vi "Striptest.vi"(1 "Simulation?":bool) -> ()   [LabVIEW 2018]
uses:
  general_VIs/globals/QC_RunInformation.vi
  striptest/ProbePlan/ProbePlanParams.vi
  InstrControl/SupplyControl/SupplyControl.lvclass
  <vilib>/regexp/Match Regular Expression.xnode
  InstrControl/InstrumentSetup.vi
  InstrControl/InstrControl.lvclass
  InstrControl/ArduinoControl/ArduinoControl.lvclass
  general_VIs/globals/QC_MeasurementSetup.vi
  InstrControl/Switching/Switching.lvclass
  InstrControl/ProbeStationControl/ProbeStationControl.lvclass
  <vilib>/Analysis/NI_AALBase.lvlib
  InstrControl/LCRControl/LCRControl.lvclass
panel:
  out "Resistance [MW]":cluster{u32, i32, "Array OUT":dbl[]}(graph)
  out "Tab Control":enum32{"Striptest Setup", "Striptest"}(tab)
  in  "Length1":dbl=2.386 caption="Length [cm]"
  in  "Length2":dbl=2.386
  in  "Length3":dbl=2.386
  in  "Length4":dbl=2.386
  in  "Bias Voltage [V]":dbl=-150.0 format="%.1f"
  in  "Frequency [Hz] Setup":i32=1000 caption="Frequency [Hz]" format="%#.3p"
  in  "Minimum fraction\nof good strips":dbl=98.0 format="%.1g"
  in  "Quit":bool
  in  "Continue":bool
  in  "Measurement Configurations":bool
  in  "Pinholes Y/N":bool=TRUE
  in  "Capacitance Y/N":bool=TRUE
  in  "Resistance Y/N":bool=TRUE
  in  "Striptest SMU":string(combo)="Keithley 2410"
  in  "LCR Meter":string(combo)="WayneKerr 6440B"
  in  "Temperature":enum16{"Read Arduino", "Enter manually"}(ring)
  in  "Bias Supply":string(combo)="Keithley 2410"
  in  "Hardware Configurations":bool
  in  "DB Serial No. IN:":string caption="DB Serial No.:"
  in  "User:":string(combo)="Christoph"
  in  "Batch No. IN:":string caption="Batch No.:"
  in  "Device Category IN:":string(combo)="Short Strip" caption="Device Category:"
  in  "Wafer No. IN:":string caption="Wafer No.:"
  in  "From4":u16(ring)
  in  "From3":u16(ring)
  in  "From2":u16(ring)
  in  "From 1":u16(ring) caption="From"
  in  "To4":u16(ring)
  in  "To3":u16(ring)
  in  "To2":u16(ring)
  in  "To 1":u16(ring) caption="To"
  out "Region 1":string caption="Region"
  out "Region2":string
  out "Region3":string
  out "Region4":string
  in  "Enable1":bool
  in  "Enable4":bool
  in  "Enable2":bool
  in  "Enable3":bool
  in  "Pinhole Parameters IN":T1={"Base Voltage"=10.0, "Base Ramp [V/step]"=10.0, "Base Step [ms]"=1000, "High Voltage"=100.0, "High Ramp [V/step]"=100.0, "High Step [ms]"=1000} caption="Pinhole Measurement Parameters"
  in  "Manufacturer:":string(combo)="Hamamatsu"
  in  "Auto ReCheck":bool
  in  "Thresholds:":T2={"Current [nA]"=200.0, "Ccoupl Lo [pF/cm]"=20.0, "Ccoupl Hi [pF/cm]"=33.0, "Rbias Lo [MW]"=1.0, "Rbias Hi [MW]"=2.0}
  in  "Rolling\nCurrent Readout":bool=TRUE
  in  "settling\ndelay [ms]":i32=50
  in  "Pinhole Parameters":T1={"Base Voltage"=10.0, "Base Ramp [V/step]"=10.0, "Base Step [ms]"=1000, "High Voltage"=100.0, "High Ramp [V/step]"=100.0, "High Step [ms]"=1000}
  out "Bias On/Off:":bool
  in  "Auto quit &\nswitch off bias":bool
  out "Sensor No.:":string
  out "Device Category:":string
  out "DB Serial No.:":string
  out "Initiated:":string
  in  "ReCheck":bool
  in  "Save Data":bool
  in  "Abort":bool
  in  "Quit w/o saving":bool
  out "Probing Region:":string
  out "Probe Point:":string
  out "Current [nA]:":dbl format="%#.2g"
  out "Capacitance [pF]:":dbl format="%#.2g"
  out "Reistance [MW]:":dbl format="%#.3g"
  out "Last Probe at:":string
  out "Run Duration:":string
  out "Estimated Completion:":string
  out "Status:":string
  out "Probe Card Channels":i32=32
  in  "Show:":u16(ring) items=["Segment4"]
  out "Defects":i32[][](graph)
  out "% OK:":dbl
  out "# total defects:":i32
  out "# probed":i32
  out "Bad Strip List":i32[](array[numeric])
  out "defect type array":i32[](array[numeric])
  out "Capacitance [pF]":cluster{u32, i32, "Array OUT":dbl[]}(graph)
  out "Current [nA]":cluster{u32, i32, "Array OUT":dbl[]}(graph)
  out "Current Reference 100V":dbl[](array[numeric])
  out "Current Reference 10V":dbl[](array[numeric])
  out "Single Needle":bool
  out "Z profile":i32[][](array[numeric])
  out "Start Temperature [°C]":dbl
  out "Last Temperature [°C]":dbl
  out "disabled channels":i32[](array[numeric])
  out "Module failed/passed":bool
  out "min scale array":i32[](array[numeric])
  out "max scale array":i32[](array[numeric])
  out "total strip number":u32
  out "Region Indices":i32[](array[numeric])
  out "Current Bias Voltage [V]":dbl
  out "Temperature Progression":T3
  out "probe points per region":i32[](array[numeric])
  # "Sensor QC: Striptest"
  # "University of \nCambridge"
  # "Current [nA]"
  # "Statistical information:"
  # "Pinholes:"
  # "Capacitance [pF]"
  # "Punchthroughs:"
  # "Shorts:"
  # "Opens:"
  # "Rpoly:"
  # "Resistance [MW]"
  # "Implant:"
  # "Current segment:"
  # "Ok  Pinhole at base  Pinhole after ramp  Short  Open  Rbias"
  # "Probe Range"
  # "Measurement Configuration"
  # "Hardware"
  # "DUT Description"
  # "Tests Included"
  # "Current status:"
  # "Measurement parameters:"
  # "DUT & Test Description:"
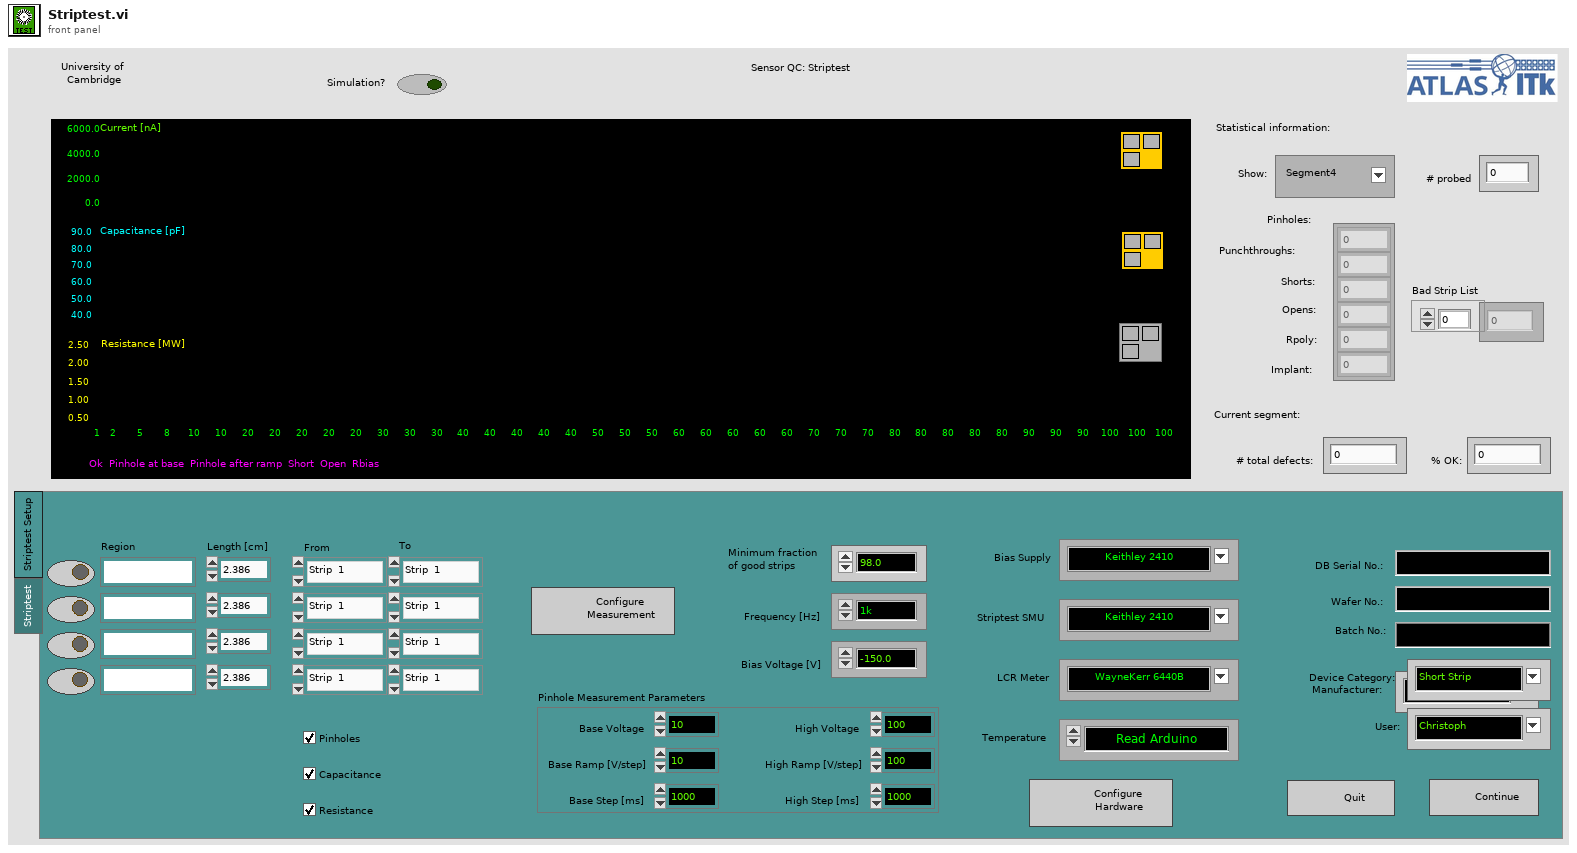
[diagram p1: front panel]
types:
  T1 = cluster{"Base Voltage":dbl, "Base Ramp [V/step]":dbl, "Base Step [ms]":i32, "High Voltage":dbl, "High Ramp [V/step]":dbl, "High Step [ms]":i32}
  T2 = cluster{"Current [nA]":dbl, "Ccoupl Lo [pF/cm]":dbl, "Ccoupl Hi [pF/cm]":dbl, "Rbias Lo [MW]":dbl, "Rbias Hi [MW]":dbl}
  T3 = cluster{"Time Array":string[], "Temperature Array [°C]":dbl[], "Humidity Array [RH %]":dbl[]}
  T4 = enum16{"Supply", "LCR", "Multimeter", "Switching"}
  T5 = enum16{"Reset", "Read Array", "Read Element", "Write Element", "Write Array", "Add Element", "Add Array"}
  T6 = enum16{"Reset", "Ground", "Striptest SMU", "Striptest LCR", "IV", "CV", "Interstrip Cap", "Interstrip Res"}
  T7 = enum16{"Reference measurement", "Baseline correcetion 10V", "Baseline correcetion 100V", "Nothing"}
  T8 = cluster{"Bias Supply":refnum<class "SupplyControl.lvclass">, "SMU":refnum<class "SupplyControl.lvclass">, "LCR":refnum<class "LCRControl.lvclass">, "ProbeStation":refnum<class "ProbeStationControl.lvclass">, "Arduino":refnum<class "ArduinoControl.lvclass">, "Measurement switch":refnum<class "Switching.lvclass">, "Probe Card Channels":i32, "Bias Voltage [V]":dbl, "First strip":i32, "Last strip":i32, "Base Voltage [V]":dbl, "Base Ramp Step [V]":dbl, "Base Ramp Interval [ms]":u32, "High Voltage [V]":dbl, "High Ramp Step [V]":dbl, "High Ramp Interval [ms]":u32, "AC frequency [Hz]":i32, "AC amplitude [V]":dbl, "RC Configuration":u16, "Single Needle":bool, "Temperature Readout":enum16{"Read Arduino", "Enter manually"}, "Fraction of good strips [%]":dbl, "Measurement switch used?":bool, "Matrix X Channels":cluster{"Mux1 C1":i32, "Mux1 C2":i32, "Mux2 C1":i32, "Mux2 C2":i32}, "Pinholes Y/N":bool, "Capacitance Y/N":bool, "Resistance Y/N":bool, "Bias Supply Name":string, "SMU Name":string, "LCR Name":string}
  T9 = cluster{"Institute":string, "Manufacturers":string[], "Devices":string[], "Serialnumbers Lookup DB":string, "Data directory":string, "Backup & screenshot directory":string, "List of known users":string[], "Measurement switch not used":bool, "Measurement Switch":string, "DUT Switch":string, "Rseries IV [MOhm]":string, "Rshunt IV [MOhm]":string, "Rseries CV [MOhm]":string, "DC blocking Cap [µF]":string, "Rseries LCR [MOhm]":string, "Rseries stability [MOhm]":string, "Rshunt stability [MOhm]":string, "Rseries striptest bias [MOhm]":string, "Rseries strip pinhole [MOhm]":string}
  T10 = cluster{"Sensor Serial No.:":string, "Wafer:":string, "Batch:":string, "Manufacturer:":string, "Device Category:":string, "Database Serial No.:":string, "Date Initiated:":string, "Time Initiated:":string, "Test":string, "Probeplan used:":string, "End of Run Status":dbl, "End of Run comment:":string, "User:":string, "Vbias SMU":string, "LCR":string, "Test SMU":string, "Test DMM":string, "Comments":string, "Measurement results":cluster{"IV":string, "CV":string, "Cis":string, "Ris":string, "Stability":string, "PTP":string, "Striptest":string}}
  T11 = cluster{"Strip Number OUT":i32, "X0":i32, "Y0":i32, "X1":i32, "Y1":i32, "Xref":dbl, "Yref":dbl, "ProbePlan type":u32, "Inner pads offset":ext, "Outer pads offset":ext, "l_inner":ext, "l_outer":ext, "strip numbering":u16, "Device Orientation":ext, "Stagger offset":i32, "Yoffset":dbl, "Strip pitch":dbl, "Fiducail separation":dbl, "Radius":ext, "Relative strip angles":dbl, "Probeplan description":string, "ProbePlan array":cluster{"Region":string, "ProbePoints":cluster{"X":dbl, "Y":dbl, "Label":string, "CardViable?":bool}[]}[], "Test ProbePoints":cluster{"Regions Enabled":bool[], "From index":u32[], "To index":u32[], "Strip length [cm]":dbl[]}}
  T12 = cluster{"Region":string, "ProbePoints":cluster{"X":dbl, "Y":dbl, "Label":string, "CardViable?":bool}[]}[]
  T13 = cluster{"VISA address":refnum<visa-resource-name>, "T sensor":enum16{"SHT", "DS"}, "Arduino":refnum<class "ArduinoControl.lvclass">}
  T14 = cluster{"X":dbl, "Y":dbl, "Label":string, "CardViable?":bool}[]
  T15 = cluster{"X":dbl, "Y":dbl, "Label":string, "CardViable?":bool}
  T16 = cluster{"pass Rate in %":dbl, "Bad channel list":i32[], "No of bad strips":i32, "Defect description list":i32[], "Number of defects per category":i32[], "Defect lists":string[], "No of channels":i32, "Defect Flag array OUT":i32[][]}
  T17 = cluster{"Hi Cap":dbl, "Lo Cap":dbl, "Current threshold":dbl, "Lo R":dbl, "Hi R":dbl}
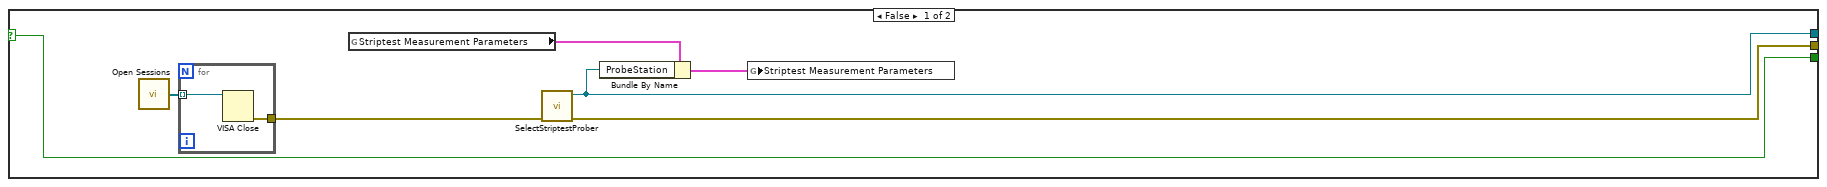
[diagram p3: hidden frame]
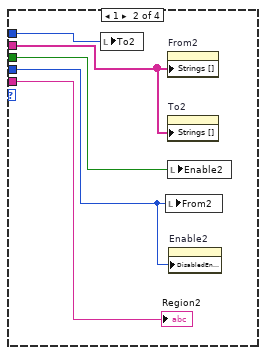
[diagram p4: hidden frame]
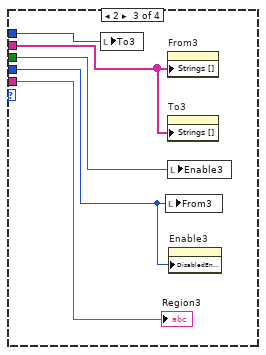
[diagram p5: hidden frame]
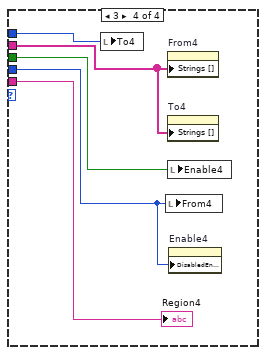
[diagram p6: hidden frame]
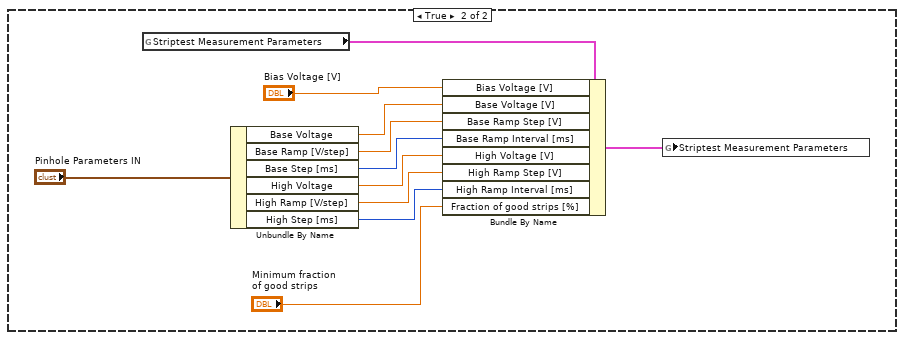
[diagram p8: hidden frame]
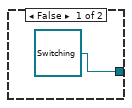
[diagram p10: hidden frame]
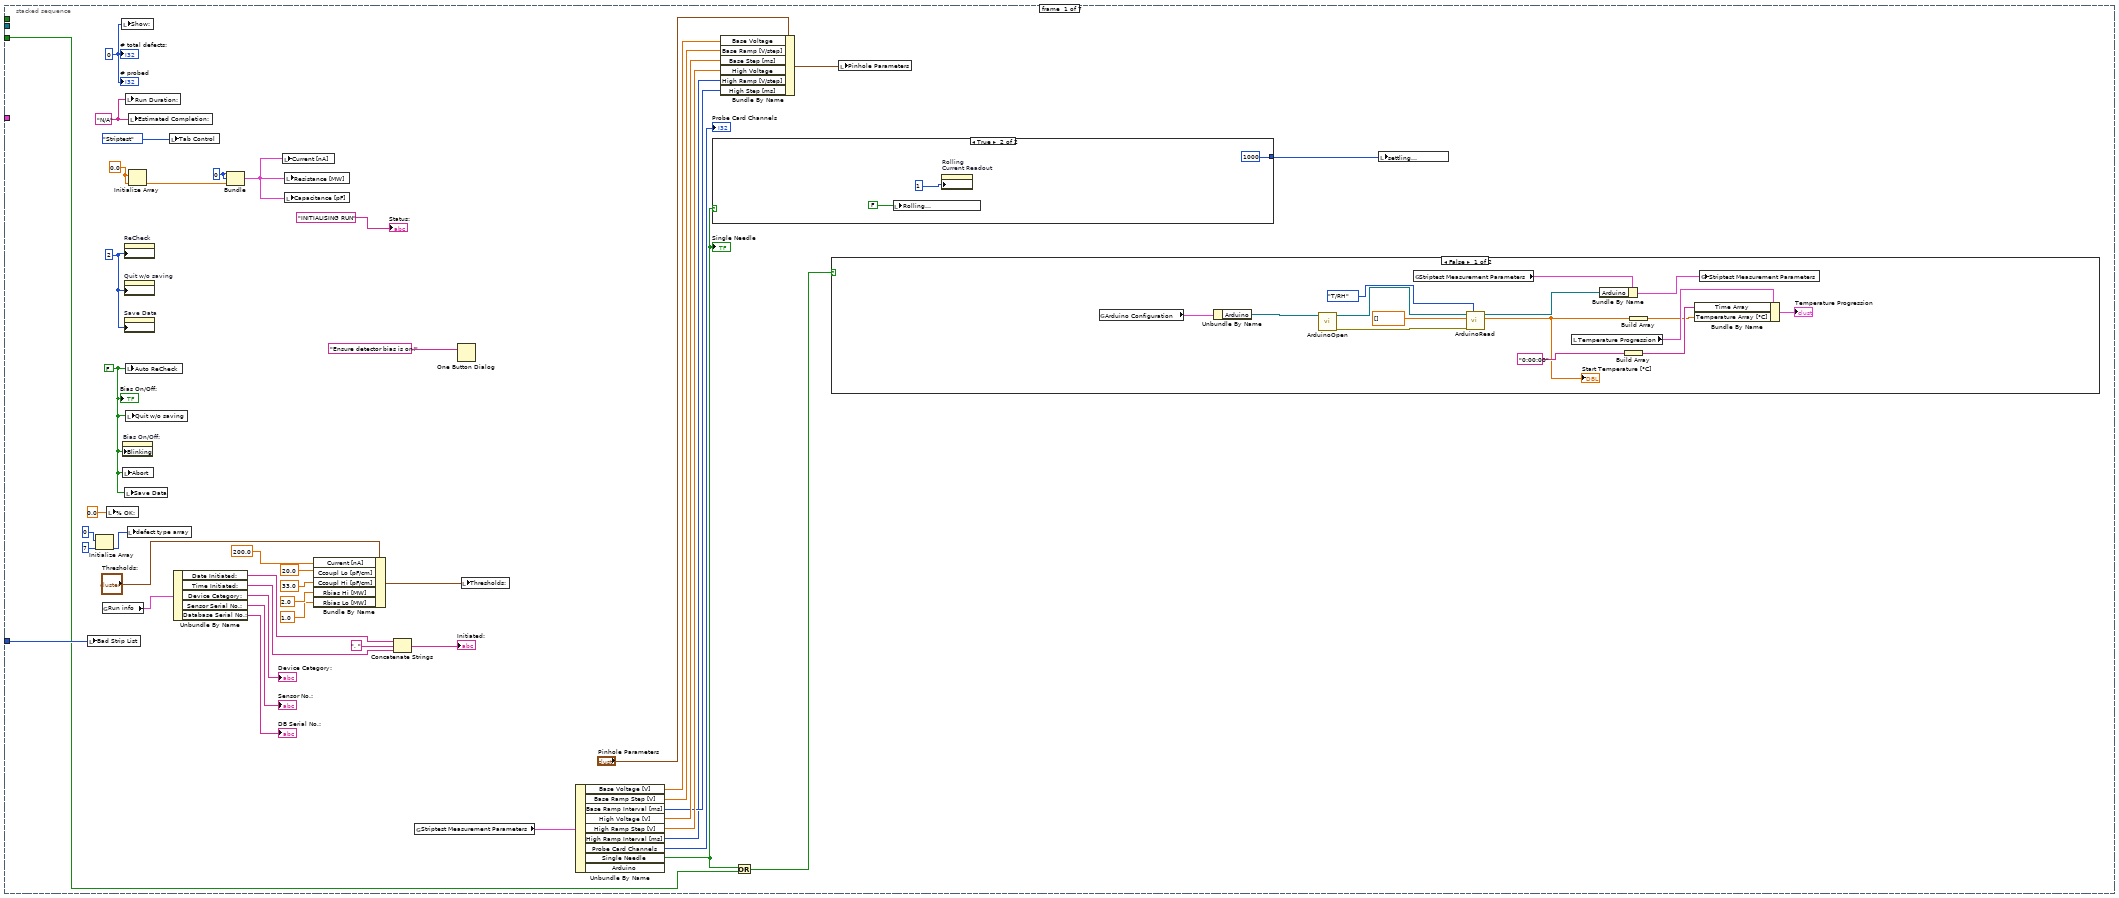
[diagram p11: hidden frame]
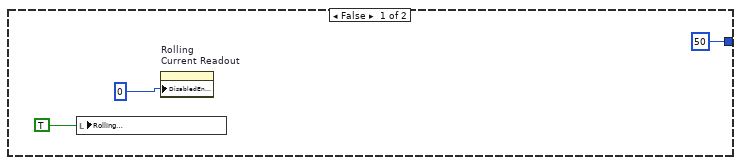
[diagram p12: hidden frame]
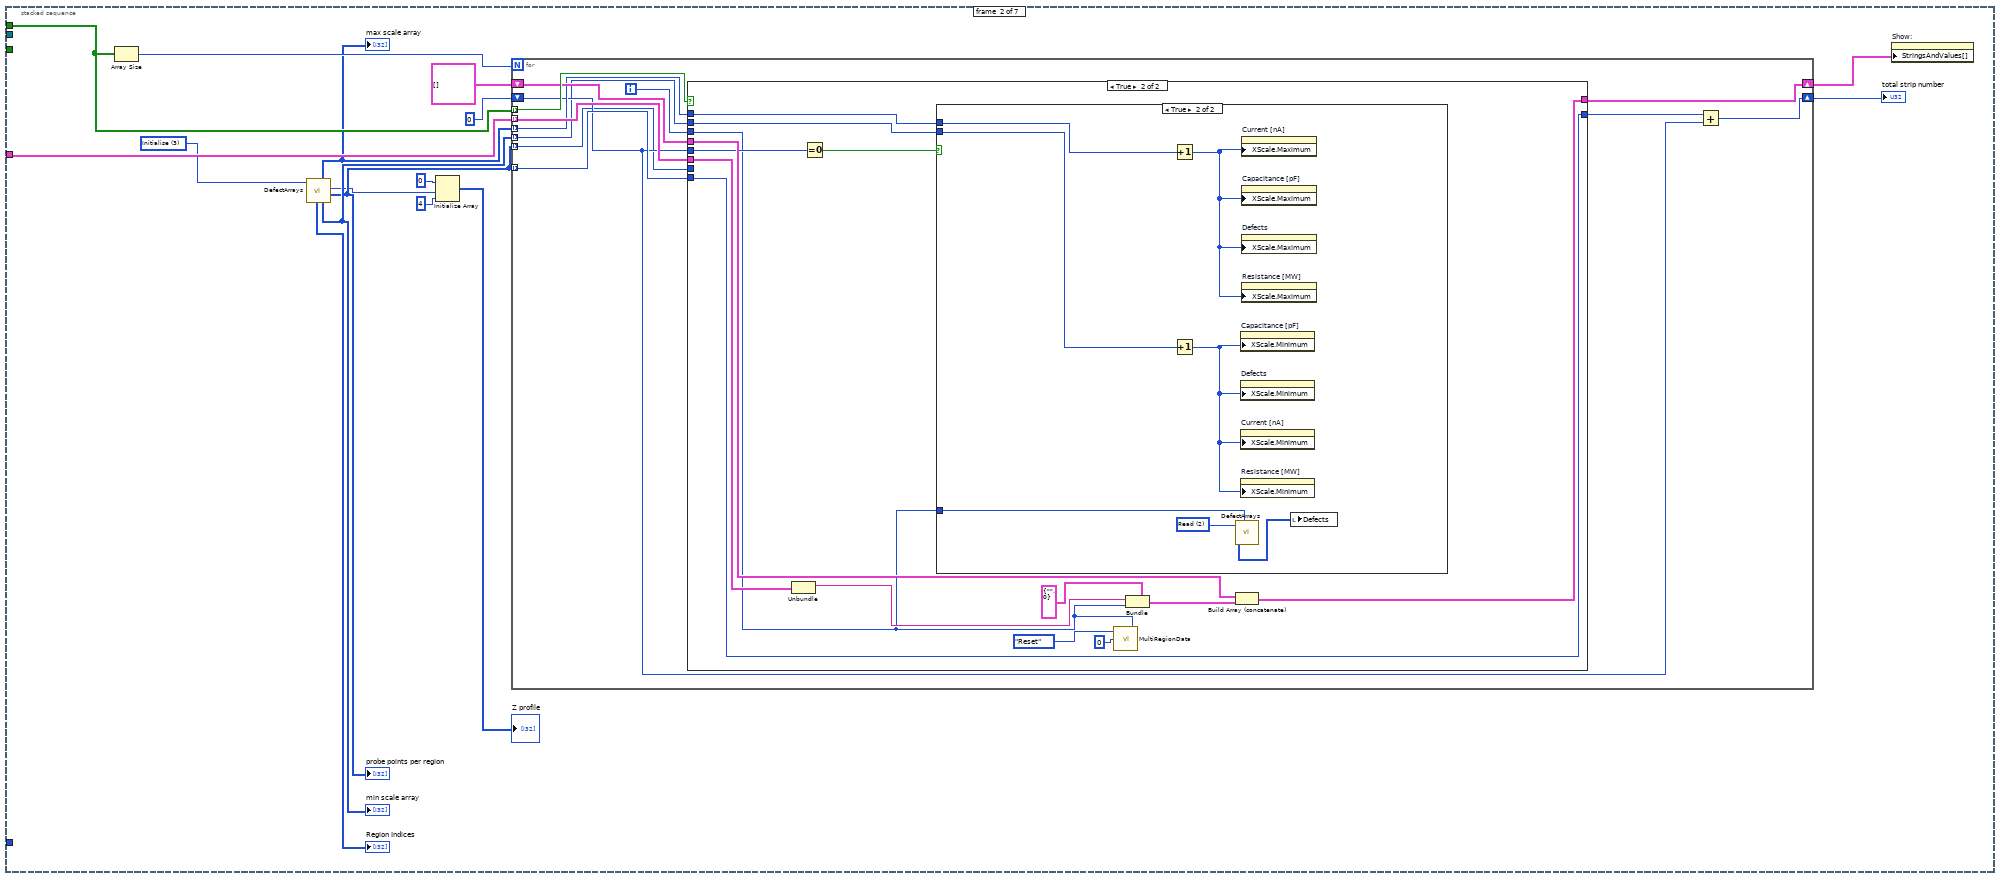
[diagram p14: hidden frame]
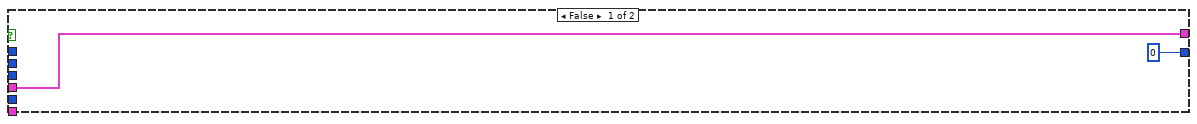
[diagram p15: hidden frame]
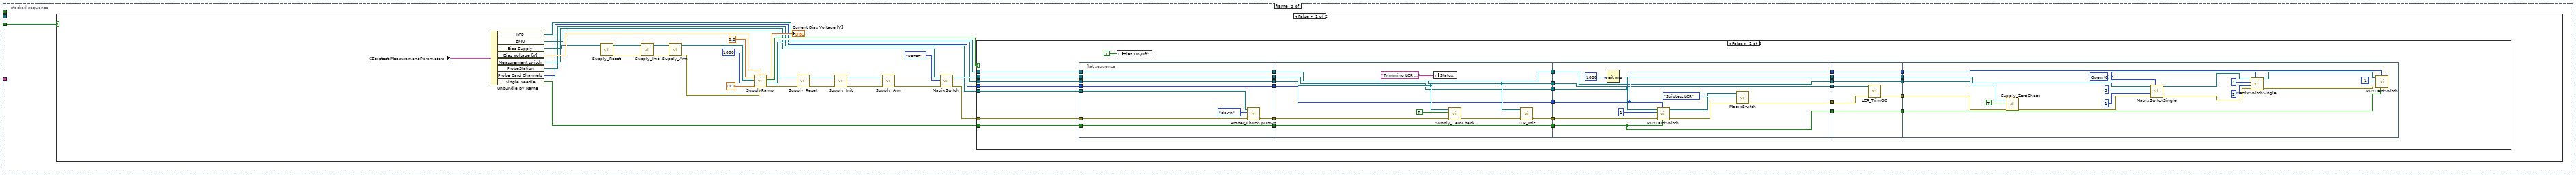
[diagram p17: hidden frame]
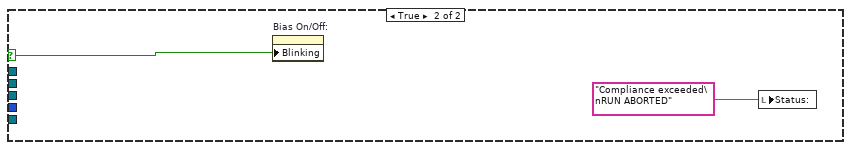
[diagram p18: hidden frame]
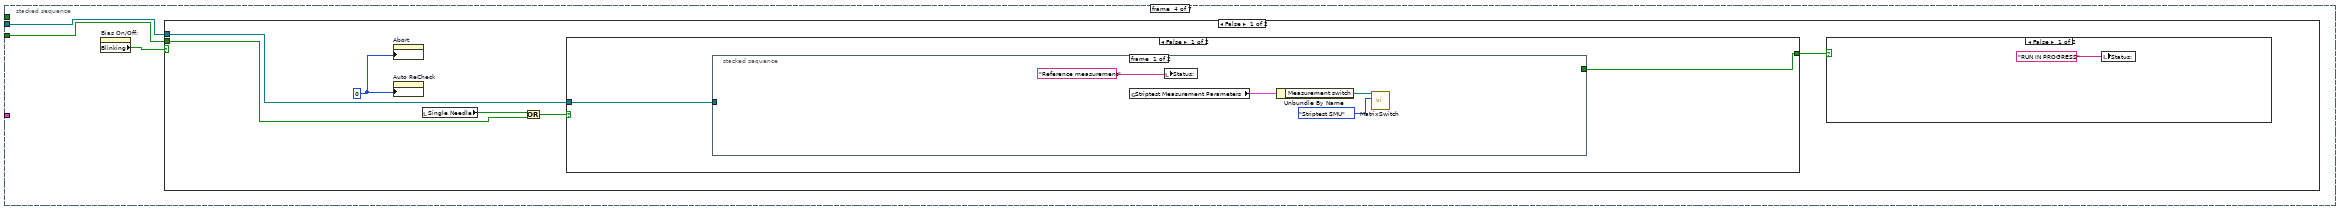
[diagram p20: hidden frame]
diagram:
  n1 = stacked-sequence {
    tunnel: "Simulation?" -> [w5 w217]
    frame #0 {
      # "Striptest setup"
      n2 = flat-sequence {
        tunnel: w5 -> [w9]
        tunnel: [w6] -> w4
        tunnel: w4 -> [w27]
        tunnel: [w27] -> w3
        tunnel: w3 -> [w103]
        tunnel: [w103] -> w2
        tunnel: w2 -> [w156]
        frame #0 {
          w12 = ""
          w13 = 2
          w14 = FALSE
          n3 = case shown="True" w9 {
            selector: w9 -> [w15 w26]
            tunnel: [w17 errorcluster {"status"=FALSE, "code"=0, "source"=""} ("error constant")] -> w8
            tunnel: [w16 refnum<class "ProbeStationControl.lvclass"> refnum ("ProbeStationControl out")] -> w7
            tunnel: [w15 w26] -> w6
            frame False {
              n4 = call <vilib>:"Open Sessions.vi"() -> ("Array of Refnums"=w19:refnum<visa-resource-name>[])  [unwired: 2 in]
              n5 = for {
                tunnel: w19 -> [w23] mode=indexing
                tunnel: [w22] -> w18
                n6 = VISA Close(VISA resource name=w23) -> (error out=w22:errorcluster)  [unwired: 1 in]
              }
              n7 = global read "QC_MeasurementSetup.vi" "Striptest Measurement Parameters"() -> (w21:T8)
              n8 = call "SelectStriptestProber.vi"("error in (no error)"=w18) -> ("error out"=w17:errorcluster, "ProbeStationControl out"=w16:refnum<class "ProbeStationControl.lvclass">)  [unwired: 9 in]
              n9 = Bundle By Name(cluster=w21, "ProbeStation"=w16) -> (w20:T8)
              n10 = global write "QC_MeasurementSetup.vi" "Striptest Measurement Parameters"(w20) -> ()
            }
            frame True {
            }
          }
          n11 = local write "Region 1"(w12) -> ()
          n12 = local write "Region2"(w12) -> ()
          n13 = local write "Region3"(w12) -> ()
          n14 = local write "Region4"(w12) -> ()
          n15 = local write "Enable2"(w14) -> ()
          n16 = local write "Enable1"(w14) -> ()
          n17 = local write "Enable3"(w14) -> ()
          n18 = local write "Enable4"(w14) -> ()
          n19 = property on="Enable4" class="Bool (strict)"("DisabledEnum"=w13) -> ()  [unwired: 2 in, 2 out]
          n20 = property on="Enable1" class="Bool (strict)"("DisabledEnum"=w13) -> ()  [unwired: 2 in, 2 out]
          n21 = property on="Enable2" class="Bool (strict)"("DisabledEnum"=w13) -> ()  [unwired: 2 in, 2 out]
          n22 = property on="Enable3" class="Bool (strict)"("DisabledEnum"=w13) -> ()  [unwired: 2 in, 2 out]
          n23 = call "GetGlobalDefaultConfiguration.vi"("Read defaults?"=TRUE) -> ()  [unwired: 3 in]
          n24 = call "GetLocalConfiguration.vi"() -> ()  [unwired: 3 in, 1 out]
          n25 = call "InitialiseProbeplan.vi"("error in (no error)"=w8, "Simulation"=w6, "ProbeStationControl in"=w7) -> ()  [unwired: 7 in, 2 out]
          "Tab Control" <- enum32{"Striptest Setup", "Striptest"}."Striptest Setup" ("Tab Control")
        }
        frame #1 {
          n26 = flat-sequence {
            frame #0 {
              n27 = call "SerialNo.vi"("DB serial number IN"="", "Run uninterrupted?"=FALSE) -> ()  [unwired: 6 in, 2 out]
              n28 = global read "QC_RunInformation.vi" "LocalConfiguration"() -> (w63:T9)
              n29 = Unbundle By Name(w63) -> ("List of known users"=w65:string[], "Devices"=w60:string[], "Manufacturers"=w59:string[])
              n30 = property on="Device Category IN:" class="CmbBox"("Strings[]"=w60) -> ()  [unwired: 2 in, 2 out]
              n31 = property on="Manufacturer:" class="CmbBox"("Strings[]"=w59) -> ()  [unwired: 2 in, 2 out]
              n32 = Index Array(array=w60, index=0) -> (element=w57:string)
              n33 = Index Array(array=w59, index=0) -> (element=w58:string)
              n34 = local write "Manufacturer:"(w58) -> ()
              n35 = property on="User:" class="CmbBox"("Strings[]"=w65, "AllowUndefStrs"=TRUE) -> ()  [unwired: 2 in, 2 out]
              n36 = local write "Device Category IN:"(w57) -> ()
            }
            frame #1 {
              n37 = global read "QC_RunInformation.vi" "Run info"() -> (w68:T10)
              n38 = Unbundle By Name(w68) -> ("Wafer:"=w69:string, "Batch:"=w70:string, "Manufacturer:"=w71:string, "Device Category:"=w72:string, "Database Serial No.:"=w73:string)
              n39 = local write "Manufacturer:"(w71) -> ()
              n40 = local write "Batch No. IN:"(w70) -> ()
              n41 = local write "Wafer No. IN:"(w69) -> ()
              n42 = local write "DB Serial No. IN:"(w73) -> ()
              n43 = local write "Device Category IN:"(w72) -> ()
            }
          }
          n44 = global read "QC_RunInformation.vi" "Run info"() -> (w47:T10)
          n45 = call "InstrumentNames.vi"("Instrument type"=T4."Supply") -> ("error out"=w50:errorcluster, "Instrument names"=w52:string[])  [unwired: 9 in]
          n46 = global read "ProbePlanParams.vi" "ProbePlan Parameters IN"() -> (w56:T11)
          n47 = Bundle By Name(cluster=w47, "Test"="STRIPTEST") -> (w48:T10)
          n48 = property on="Bias Supply" class="CmbBox"("Strings[]"=w52) -> ()  [unwired: 2 in, 2 out]
          n49 = property on="Striptest SMU" class="CmbBox"("Strings[]"=w52) -> ()  [unwired: 2 in, 2 out]
          n50 = global write "QC_RunInformation.vi" "Run info"(w48) -> ()
          n51 = call "InstrumentNames.vi"("error in (no error)"=w50, "Instrument type"=T4."LCR") -> ("Instrument names"=w49:string[])  [unwired: 8 in, 1 out]
          n52 = global read "QC_MeasurementSetup.vi" "Striptest Measurement Parameters"() -> (w46:T8)
          n53 = property on="LCR Meter" class="CmbBox"("Strings[]"=w49) -> ()  [unwired: 2 in, 2 out]
          n54 = Unbundle By Name(w56) -> ("ProbePlan array"=w55:T12)
          n55 = Array Size(array=w55) -> (size(s)=w54:i32)
          n56 = for {
            N: w54 -> [_]
            tunnel: w55 -> [w75]
            tunnel: w55 -> [w79] mode=indexing
            i -> [w82]
            n57 = Unbundle(w79) -> ("Region"=w78:string)  [unwired: 1 out]
            n58 = call "GetLabels.vi"("Array"=w75) -> ("Strip Labels"=w74:string[])  [unwired: 3 out]
            n59 = Array Size(array=w74) -> (size(s)=w77:i32)
            n60 = Decrement(x=w77) -> (x-1=w76:i32)
            n61 = case shown="0, Default" w82 {
              tunnel: TRUE -> [w87 w91 w97 w102]
              tunnel: 0 -> [w83 w89 w93 w99]
              tunnel: w78 -> [w85 w90 w95 w100]
              tunnel: w74 -> [w84 w88 w94 w98]
              tunnel: w76 -> [w86 w92 w96 w101]
              frame 0, Default {
                n62 = local write "To 1"(w86) -> ()
                n63 = local write "From 1"(w83) -> ()
                n64 = property on="To 1" class="Ring (strict)"("Strings []"=w84) -> ()  [unwired: 2 in, 2 out]
                n65 = property on="From 1" class="Ring (strict)"("Strings []"=w84) -> ()  [unwired: 2 in, 2 out]
                n66 = local write "Enable1"(w87) -> ()
                n67 = property on="Enable1" class="Bool (strict)"("DisabledEnum"=w83) -> ()  [unwired: 2 in, 2 out]
                "Region 1" <- w85
              }
              frame 1 {
                n68 = local write "To2"(w92) -> ()
                n69 = local write "From2"(w89) -> ()
                n70 = property on="From2" class="Ring (strict)"("Strings []"=w88) -> ()  [unwired: 2 in, 2 out]
                n71 = property on="To2" class="Ring (strict)"("Strings []"=w88) -> ()  [unwired: 2 in, 2 out]
                n72 = local write "Enable2"(w91) -> ()
                n73 = property on="Enable2" class="Bool (strict)"("DisabledEnum"=w89) -> ()  [unwired: 2 in, 2 out]
                "Region2" <- w90
              }
              frame 2 {
                n74 = local write "To3"(w96) -> ()
                n75 = local write "From3"(w93) -> ()
                n76 = property on="From3" class="Ring (strict)"("Strings []"=w94) -> ()  [unwired: 2 in, 2 out]
                n77 = property on="To3" class="Ring (strict)"("Strings []"=w94) -> ()  [unwired: 2 in, 2 out]
                n78 = local write "Enable3"(w97) -> ()
                n79 = property on="Enable3" class="Bool (strict)"("DisabledEnum"=w93) -> ()  [unwired: 2 in, 2 out]
                "Region3" <- w95
              }
              frame 3 {
                n80 = local write "To4"(w101) -> ()
                n81 = local write "From4"(w99) -> ()
                n82 = property on="From4" class="Ring (strict)"("Strings []"=w98) -> ()  [unwired: 2 in, 2 out]
                n83 = property on="To4" class="Ring (strict)"("Strings []"=w98) -> ()  [unwired: 2 in, 2 out]
                n84 = local write "Enable4"(w102) -> ()
                n85 = property on="Enable4" class="Bool (strict)"("DisabledEnum"=w99) -> ()  [unwired: 2 in, 2 out]
                "Region4" <- w100
              }
            }
          }
          n86 = Unbundle By Name(w46) -> ("Probe Card Channels"=w45:i32, "Bias Voltage [V]"=w36:dbl, "Base Voltage [V]"=w42:dbl, "Base Ramp Step [V]"=w41:dbl, "Base Ramp Interval [ms]"=w40:u32, "High Voltage [V]"=w39:dbl, "High Ramp Step [V]"=w38:dbl, "High Ramp Interval [ms]"=w37:u32, "Single Needle"=w35:bool, "Temperature Readout"=w34:enum16{"Read Arduino", "Enter manually"}, "Fraction of good strips [%]"=w33:dbl, "AC frequency [Hz]"=w32:i32, "Pinholes Y/N"=w31:bool, "Capacitance Y/N"=w30:bool, "Resistance Y/N"=w29:bool)
          n87 = local read "Pinhole Parameters IN"() -> (w44:T1)
          n88 = local write "Temperature"(w34) -> ()
          n89 = local write "Pinholes Y/N"(w31) -> ()
          n90 = local write "Single Needle"(w35) -> ()
          n91 = local write "Resistance Y/N"(w29) -> ()
          n92 = local write "Capacitance Y/N"(w30) -> ()
          n93 = local write "Bias Voltage [V]"(w36) -> ()
          n94 = Bundle By Name(cluster=w44, "Base Voltage"=w42, "Base Ramp [V/step]"=w41, "Base Step [ms]"=w40, "High Voltage"=w39, "High Ramp [V/step]"=w38, "High Step [ms]"=w37) -> (w43:T1)
          n95 = local write "Probe Card Channels"(w45) -> ()
          n96 = local write "Frequency [Hz] Setup"(w32) -> ()
          n97 = local write "Minimum fraction\nof good strips"(w33) -> ()
          n98 = local write "Pinhole Parameters IN"(w43) -> ()
        }
        frame #2 {
          n99 = while {
            shift-right: [w107] -> _
            shift-left: FALSE -> [w109]
            stop <- "Continue" stop-if-true
            n100 = Stop(stop? (T)="Quit") -> ()
            n101 = local read "DB Serial No. IN:"() -> (w113:string)
            n102 = local read "Wafer No. IN:"() -> (w115:string)
            n103 = local read "Batch No. IN:"() -> (w114:string)
            n104 = Empty String/Path?(string/path=w115) -> (empty?=w112:bool)
            n105 = Empty String/Path?(string/path=w114) -> (empty?=w111:bool)
            n106 = Empty String/Path?(string/path=w113) -> (empty?=w110:bool)
            n107 = case shown="True" "Measurement Configurations" {
              frame False {
              }
              frame True {
                n108 = Two Button Dialog(message="With this, you will change QC measurement parameters defined by the collaboration!\n\nDo you really wish to continue?", 2:"YES") -> (T button?=w121:bool)  [unwired: 1 in]
                n109 = case shown="False" w121 {
                  frame False {
                    n110 = global read "QC_MeasurementSetup.vi" "Striptest Measurement Parameters"() -> (w134:T8)
                    n111 = Unbundle By Name(w134) -> ("Bias Voltage [V]"=w124:dbl, "Base Voltage [V]"=w131:dbl, "Base Ramp Step [V]"=w130:dbl, "Base Ramp Interval [ms]"=w129:u32, "High Voltage [V]"=w128:dbl, "High Ramp Step [V]"=w127:dbl, "High Ramp Interval [ms]"=w126:u32, "Fraction of good strips [%]"=w125:dbl)
                    n112 = local read "Pinhole Parameters IN"() -> (w133:T1)
                    n113 = local write "Bias Voltage [V]"(w124) -> ()
                    n114 = Bundle By Name(cluster=w133, "Base Voltage"=w131, "Base Ramp [V/step]"=w130, "Base Step [ms]"=w129, "High Voltage"=w128, "High Ramp [V/step]"=w127, "High Step [ms]"=w126) -> (w132:T1)
                    n115 = local write "Minimum fraction\nof good strips"(w125) -> ()
                    n116 = local write "Pinhole Parameters IN"(w132) -> ()
                  }
                  frame True {
                    n117 = global read "QC_MeasurementSetup.vi" "Striptest Measurement Parameters"() -> (w145:T8)
                    n118 = Unbundle By Name("Pinhole Parameters IN") -> ("Base Voltage"=w141:dbl, "Base Ramp [V/step]"=w140:dbl, "Base Step [ms]"=w139:i32, "High Voltage"=w138:dbl, "High Ramp [V/step]"=w137:dbl, "High Step [ms]"=w136:i32)
                    n119 = Bundle By Name(cluster=w145, "Bias Voltage [V]"="Bias Voltage [V]", "Base Voltage [V]"=w141, "Base Ramp Step [V]"=w140, "Base Ramp Interval [ms]"=w139, "High Voltage [V]"=w138, "High Ramp Step [V]"=w137, "High Ramp Interval [ms]"=w136, "Fraction of good strips [%]"="Minimum fraction\nof good strips") -> (w144:T8)
                    n120 = global write "QC_MeasurementSetup.vi" "Striptest Measurement Parameters"(w144) -> ()
                  }
                }
              }
            }
            n121 = case shown="True" "Hardware Configurations" {
              tunnel: [w146 w147] -> w107
              tunnel: w109 -> [w146 _]
              frame False {
              }
              frame True {
                n122 = call "HardwareConfiguration.vi"() -> ("configured?"=w147:bool)  [unwired: 11 in]
              }
            }
            n123 = Compound Arithmetic op=OR(w112, w111, w110) -> (invert w116:bool)
            n124 = Select(t=0, s=w116, f=2) -> (s? t:f=w106:i32)
            n125 = property on="Continue" class="Bool"("DisabledEnum"=w106) -> ()  [unwired: 2 in, 2 out]
          }
        }
        frame #3 {
          w183 = T4."Supply" ("Instrument type")
          n126 = Not(x=w156) -> (.not. x?=w155:bool)
          n127 = global read "QC_RunInformation.vi" "LocalConfiguration"() -> (w162:T9)
          n128 = call "InstrumentSelection.vi"("Verify GPIB address"=w155, "Instrument type"=w183, "Instrument name IN"="Bias Supply") -> ("error out"=w189:errorcluster, "Instrument name OUT"=w164:string, "Supply"=w184:refnum<class "SupplyControl.lvclass">)  [unwired: 3 in, 3 out]
          n129 = call "InstrumentSelection.vi"("error in (no error)"=w189, "Verify GPIB address"=w155, "Instrument type"=w183, "Instrument name IN"="Striptest SMU") -> ("error out"=w179:errorcluster, "Instrument name OUT"=w163:string, "Supply"=w181:refnum<class "SupplyControl.lvclass">)  [unwired: 2 in, 3 out]
          n130 = Unbundle By Name(w162) -> ("Measurement Switch"=w161:string, "Measurement switch not used"=w160:bool)
          n131 = global read "ProbePlanParams.vi" "ProbePlan Parameters IN"() -> (w210:T11)
          n132 = Build Array("Enable1", "Enable2", "Enable3", "Enable4") -> (w208:bool[])
          n133 = Build Array("From 1", "From2", "From3", "From4") -> (w207:u16[])
          n134 = Build Array("To 1", "To2", "To3", "To4") -> (w206:u16[])
          n135 = Build Array("Length1", "Length2", "Length3", "Length4") -> (w148:dbl[])
          n136 = Bundle By Name(cluster=w210, "Test ProbePoints.Regions Enabled"=w208, "Test ProbePoints.From index"=w207, "Test ProbePoints.To index"=w206, "Test ProbePoints.Strip length [cm]"=w148) -> (w209:T11)
          n137 = Unbundle By Name(w210) -> ("Probeplan description"=w176:string)
          n138 = Concatenate Strings("Batch No. IN:", "-", "Wafer No. IN:") -> (w168:string)
          n139 = call "InstrumentSelection.vi"("error in (no error)"=w179, "Verify GPIB address"=w155, "Instrument type"=T4."LCR", "Instrument name IN"="LCR Meter") -> ("error out"=w159:errorcluster, "Instrument name OUT"=w165:string, "LCR"=w180:refnum<class "LCRControl.lvclass">)  [unwired: 2 in, 3 out]
          n140 = Not(x=w160) -> (.not. x?=w157:bool)
          n141 = global read "QC_RunInformation.vi" "Run info"() -> (w187:T10)
          n142 = case shown="True" w157 {
            tunnel: w159 -> [_ w215]
            tunnel: [refnum<class "Switching.lvclass"> refnum ("Switching") w214] -> w158
            tunnel: w155 -> [_ w213]
            tunnel: w161 -> [_ w212]
            frame False {
            }
            frame True {
              n143 = call "InstrumentSelection.vi"("error in (no error)"=w215, "Verify GPIB address"=w213, "Instrument type"=T4."Switching", "Instrument name IN"=w212) -> ("Switching"=w214:refnum<class "Switching.lvclass">)  [unwired: 2 in, 5 out]
            }
          }
          n144 = call "DateTime_OS-indep.vi"() -> ("Time"=w153:string, "Date"=w154:string)
          n145 = global write "ProbePlanParams.vi" "ProbePlan Parameters IN"(w209) -> ()
          n146 = Bundle By Name(cluster=w187, "Sensor Serial No.:"=w168, "Wafer:"="Wafer No. IN:", "Batch:"="Batch No. IN:", "Manufacturer:"="Manufacturer:", "Device Category:"="Device Category IN:", "Database Serial No.:"="DB Serial No. IN:", "Date Initiated:"=w154, "Time Initiated:"=w153, "Vbias SMU"=w164, "LCR"=w165, "Test SMU"=w163, "Probeplan used:"=w176, "User:"="User:") -> (w193:T10)
          n147 = global write "QC_RunInformation.vi" "Run info"(w193) -> ()
          n148 = global read "QC_MeasurementSetup.vi" "Striptest Measurement Parameters"() -> (w186:T8)
          n149 = Bundle By Name(cluster=w186, "Bias Supply"=w184, "SMU"=w181, "LCR"=w180, "Measurement switch"=w158, "Measurement switch used?"=w157, "Temperature Readout"="Temperature", "AC frequency [Hz]"="Frequency [Hz] Setup", "Pinholes Y/N"="Pinholes Y/N", "Capacitance Y/N"="Capacitance Y/N", "Resistance Y/N"="Resistance Y/N") -> (w185:T8)
          n150 = global write "QC_MeasurementSetup.vi" "Striptest Measurement Parameters"(w185) -> ()
        }
      }
    }
    frame #1 {
      # "Striptest measurement procedure"
      n151 = global read "QC_MeasurementSetup.vi" "Striptest Measurement Parameters"() -> (w218:T8)
      n152 = global read "ProbePlanParams.vi" "ProbePlan Parameters IN"() -> (w224:T11)
      n153 = Unbundle By Name(w224) -> ("Test ProbePoints.Regions Enabled"=w221:bool[], "ProbePlan array"=w220:T12)
      n154 = Unbundle By Name(w218) -> ("ProbeStation"=w219:refnum<class "ProbeStationControl.lvclass">)
      n155 = Initialize Array(0) -> (w222:i32[])  [unwired: 1 in]
      n156 = stacked-sequence {
        tunnel: w222 -> [w249 _ _ _ w486 _ _]
        tunnel: w217 -> [w244 _ w342 w463 w485 w1108 w1170]
        tunnel: w221 -> [_ w305 _ _ w489 _ w1169]
        tunnel: w220 -> [_ w304 _ _ w487 _ _]
        tunnel: w219 -> [_ _ _ w461 _ w1109 _]
        frame #0 {
          w251 = "N/A"
          w246 = FALSE
          w259 = 2
          w252 = 0
          w268 = 0
          w267 = 0.0
          n157 = local write "Bad Strip List"(w249) -> ()
          n158 = Initialize Array(0, 7 ("Dimension Size")) -> (w247:i32[])
          n159 = global read "QC_RunInformation.vi" "Run info"() -> (w265:T10)
          n160 = local write "% OK:"(0.0) -> ()
          n161 = local write "Show:"(w252) -> ()
          n162 = local write "Abort"(w246) -> ()
          n163 = property on="Bias On/Off:" class="Bool (strict)"("Blinking"=w246) -> ()  [unwired: 2 in, 2 out]
          n164 = property on="ReCheck" class="Bool"("DisabledEnum"=w259) -> ()  [unwired: 2 in, 2 out]
          n165 = property on="Quit w/o saving" class="Bool (strict)"("DisabledEnum"=w259) -> ()  [unwired: 2 in, 2 out]
          n166 = property on="Save Data" class="Bool (strict)"("DisabledEnum"=w259) -> ()  [unwired: 2 in, 2 out]
          n167 = local write "Save Data"(w246) -> ()
          n168 = local write "Run Duration:"(w251) -> ()
          n169 = local write "Auto ReCheck"(w246) -> ()
          n170 = local write "Quit w/o saving"(w246) -> ()
          n171 = local write "defect type array"(w247) -> ()
          n172 = Initialize Array(w267, w267) -> (w269:dbl[])
          n173 = local write "Estimated Completion:"(w251) -> ()
          n174 = local write "Tab Control"(enum32{"Striptest Setup", "Striptest"}."Striptest" ("Tab Control")) -> ()
          n175 = Unbundle By Name(w265) -> ("Date Initiated:"=w227:string, "Time Initiated:"=w225:string, "Device Category:"=→"Device Category:":string, "Sensor Serial No.:"=→"Sensor No.:":string, "Database Serial No.:"=→"DB Serial No.:":string)
          n176 = Bundle(w268, w268, w269) -> (w266:cluster{i32, i32, dbl[]})  [unwired: 1 in]
          n177 = local write "Current [nA]"(w266) -> ()
          n178 = local write "Resistance [MW]"(w266) -> ()
          n179 = local write "Capacitance [pF]"(w266) -> ()
          n180 = Bundle By Name(cluster="Thresholds:", "Current [nA]"=200.0 ("CapLo"), "Ccoupl Lo [pF/cm]"=20.0 ("CapLo"), "Ccoupl Hi [pF/cm]"=33.0 ("CapHi"), "Rbias Hi [MW]"=2.0 ("Rpolyhi"), "Rbias Lo [MW]"=1.0 ("RpolyLo")) -> (w257:T2)
          n181 = Concatenate Strings(w227, ", ", w225) -> (→"Initiated:":string)
          n182 = global read "QC_MeasurementSetup.vi" "Striptest Measurement Parameters"() -> (w232:T8)
          n183 = One Button Dialog(message="Ensure detector bias is on!") -> ()  [unwired: 1 in, 1 out]
          n184 = local write "Thresholds:"(w257) -> ()
          n185 = Unbundle By Name(w232) -> ("Base Voltage [V]"=w240:dbl, "Base Ramp Step [V]"=w241:dbl, "Base Ramp Interval [ms]"=w237:u32, "High Voltage [V]"=w238:dbl, "High Ramp Step [V]"=w239:dbl, "High Ramp Interval [ms]"=w236:u32, "Probe Card Channels"=→"Probe Card Channels":i32, "Single Needle"=w231:bool)  [unwired: 1 out]
          "Single Needle" <- w231
          n186 = case shown="True" w231 {
            tunnel: [50 1000] -> w233
            frame False {
              n187 = local write "Rolling\nCurrent Readout"(TRUE) -> ()
              n188 = property on="Rolling\nCurrent Readout" class="Bool (strict)"("DisabledEnum"=0) -> ()  [unwired: 2 in, 2 out]
            }
            frame True {
              n189 = local write "Rolling\nCurrent Readout"(FALSE) -> ()
              n190 = property on="Rolling\nCurrent Readout" class="Bool (strict)"("DisabledEnum"=1) -> ()  [unwired: 2 in, 2 out]
            }
          }
          n191 = Bundle By Name(cluster="Pinhole Parameters", "Base Voltage"=w240, "Base Ramp [V/step]"=w241, "Base Step [ms]"=w238, "High Voltage"=w239, "High Ramp [V/step]"=w236, "High Step [ms]"=w237) -> (w242:T1)
          n192 = Or(x=w231, y=w244) -> (x .or. y?=w243:bool)
          n193 = case shown="False" w243 {
            frame False {
              n194 = global read "InstrumentSetup.vi" "Arduino Configuration"() -> (w290:T13)
              n195 = Unbundle By Name(w290) -> ("Arduino"=w282:refnum<class "ArduinoControl.lvclass">)
              n196 = call "ArduinoOpen.vi"("ArduinoControl in"=w282) -> ("error out"=w280:errorcluster, "ArduinoControl out"=w281:refnum<class "ArduinoControl.lvclass">)  [unwired: 9 in]
              n197 = global read "QC_MeasurementSetup.vi" "Striptest Measurement Parameters"() -> (w278:T8)
              n198 = call "ArduinoRead.vi"("Arduino function"=enum16{"T/RH", "Interlock", "Edgesense"}."T/RH", "error in (no error)"=w280, "Temperature IN"=dbl[] [], "ArduinoControl in"=w281) -> ("Temperature [°C]"=w284:dbl, "ArduinoControl out"=w276:refnum<class "ArduinoControl.lvclass">)  [unwired: 2 in, 4 out]
              "Start Temperature [°C]" <- w284
              n199 = local read "Temperature Progression"() -> (w289:T3)
              n200 = Bundle By Name(cluster=w278, "Arduino"=w276) -> (w277:T8)
              n201 = Build Array("0:00:00") -> (w285:string[])
              n202 = Build Array(w284) -> (w283:dbl[])
              n203 = Bundle By Name(cluster=w289, "Time Array"=w285, "Temperature Array [°C]"=w283) -> (→"Temperature Progression":T3)
              n204 = global write "QC_MeasurementSetup.vi" "Striptest Measurement Parameters"(w277) -> ()
            }
            frame True {
            }
          }
          n205 = local write "Pinhole Parameters"(w242) -> ()
          n206 = local write "settling\ndelay [ms]"(w233) -> ()
          "# total defects:" <- w252
          "# probed" <- w252
          "Status:" <- "INITIALISING RUN"
          "Bias On/Off:" <- w246
        }
        frame #1 {
          w300 = u16 3 items=["Nothing", "Write", "Read", "Initialise"] ("action")
          n207 = Array Size(array=w305) -> (size(s)=w306:i32)
          n208 = call "DefectArrays.vi"("action"=w300) -> ("Region Indices"=→"Region Indices":i32[], "To"=w299:i32[], "max. No. of points in region"=w291:i32, "From"=w298:i32[], "No. of points in region"=w293:i32[])  [unwired: 2 in, 3 out]
          "max scale array" <- w299
          "min scale array" <- w298
          "probe points per region" <- w293
          n209 = Initialize Array(0, w291, 4) -> (→"Z profile":i32[][])
          n210 = for {
            N: w306 -> [_]
            tunnel: w305 -> [w318] mode=indexing
            shift-right: [w317] -> w303
            shift-left: cluster{string, i32}[] [] -> [w316]
            tunnel: w304 -> [w315] mode=indexing
            tunnel: w293 -> [w310] mode=indexing
            tunnel: w299 -> [w311] mode=indexing
            tunnel: w298 -> [w308] mode=indexing
            shift-right: [w312] -> w302
            shift-left: 0 -> [w309]
            tunnel: w293 -> [w307] mode=indexing
            i -> [w313]
            n211 = case shown="True" w318 {
              tunnel: w316 -> [w319 w333]
              tunnel: [w319 w332] -> w317
              tunnel: w315 -> [_ w334]
              tunnel: [0 w328] -> w314
              tunnel: w313 -> [_ w325]
              tunnel: w311 -> [_ w330]
              tunnel: w308 -> [_ w329]
              tunnel: w310 -> [_ w328]
              tunnel: w309 -> [_ w327]
              tunnel: w307 -> [_ _]
              frame False {
              }
              frame True {
                n212 = Unbundle(w334) -> ("Region"=w326:string)  [unwired: 1 out]
                n213 = Equal To 0?(x=w327) -> (x = 0?=w331:bool)
                n214 = case shown="True" w331 {
                  tunnel: w330 -> [_ w336]
                  tunnel: w329 -> [_ w338]
                  tunnel: w325 -> [_ w339]
                  frame False {
                  }
                  frame True {
                    w341 = u16 2 items=["Nothing", "Write", "Read", "Initialise"] ("action")
                    n215 = Increment(x=w336) -> (x+1=w335:i32)
                    n216 = Increment(x=w338) -> (x+1=w337:i32)
                    n217 = call "DefectArrays.vi"("action"=w341, "Region Index"=w339) -> ("Defect array OUT"=w340:i32[][])  [unwired: 1 in, 7 out]
                    n218 = property on="Capacitance [pF]" class="WFGraph (strict)"("XScale.Minimum"=w337) -> ()  [unwired: 2 in, 2 out]
                    n219 = property on="Defects" class="IntGraph (strict)"("XScale.Minimum"=w337) -> ()  [unwired: 2 in, 2 out]
                    n220 = property on="Current [nA]" class="WFGraph (strict)"("XScale.Minimum"=w337) -> ()  [unwired: 2 in, 2 out]
                    n221 = property on="Resistance [MW]" class="WFGraph (strict)"("XScale.Minimum"=w337) -> ()  [unwired: 2 in, 2 out]
                    n222 = property on="Current [nA]" class="WFGraph (strict)"("XScale.Maximum"=w335) -> ()  [unwired: 2 in, 2 out]
                    n223 = property on="Capacitance [pF]" class="WFGraph (strict)"("XScale.Maximum"=w335) -> ()  [unwired: 2 in, 2 out]
                    n224 = property on="Defects" class="IntGraph (strict)"("XScale.Maximum"=w335) -> ()  [unwired: 2 in, 2 out]
                    n225 = property on="Resistance [MW]" class="WFGraph (strict)"("XScale.Maximum"=w335) -> ()  [unwired: 2 in, 2 out]
                    n226 = local write "Defects"(w340) -> ()
                  }
                }
                n227 = call "MultiRegionData.vi"("Action"=T5."Reset", "Array Size / Index"=0, "Region index"=w325) -> ()  [unwired: 3 in, 2 out]
                n228 = Bundle(cluster=cluster{string, i32} {"", 0}, w326, w325) -> (w324:cluster{string, i32})
                n229 = Build Array (concatenate)(w333, w324) -> (w332:cluster{string, i32}[])
              }
            }
            n230 = Add(x=w314, y=w309) -> (x+y=w312:i32)
          }
          "total strip number" <- w302
          n231 = property on="Show:" class="Ring (strict)"("StringsAndValues[]"=w303) -> ()  [unwired: 2 in, 2 out]
        }
        frame #2 {
          n232 = case shown="False" w342 {
            frame False {
              n233 = global read "QC_MeasurementSetup.vi" "Striptest Measurement Parameters"() -> (w371:T8)
              n234 = Unbundle By Name(w371) -> ("LCR"=w348:refnum<class "LCRControl.lvclass">, "SMU"=w349:refnum<class "SupplyControl.lvclass">, "Bias Supply"=w350:refnum<class "SupplyControl.lvclass">, "Bias Voltage [V]"=w360:dbl, "Measurement switch"=w345:refnum<class "Switching.lvclass">, "ProbeStation"=w347:refnum<class "ProbeStationControl.lvclass">, "Probe Card Channels"=w344:i32, "Single Needle"=w343:bool)
              n235 = call-dynamic "Supply_Reset.vi"("SupplyControl in"=w350) -> ("error out"=w364:errorcluster, "SupplyControl out"=w367:refnum<class "SupplyControl.lvclass">)  [unwired: 9 in]
              n236 = call-dynamic "Supply_Init.vi"("error in (no error)"=w364, "SupplyControl in"=w367) -> ("error out"=w365:errorcluster, "SupplyControl out"=w366:refnum<class "SupplyControl.lvclass">)  [unwired: 8 in]
              n237 = call-dynamic "Supply_Arm.vi"("error in (no error)"=w365, "SupplyControl in"=w366) -> ("error out"=w362:errorcluster, "SupplyControl out"=w363:refnum<class "SupplyControl.lvclass">)  [unwired: 8 in]
              n238 = call "SupplyRamp.vi"("error in"=w362, "Requested Voltage"=w360, "Step Size"=10.0, "Step Delay"=1000, "Supply IN"=w363, "Starting Voltage"=0.0) -> ("error out"=w361:errorcluster, "Supply OUT"=w346:refnum<class "SupplyControl.lvclass">, "Compliance exceeded"=w354:bool, "Current Voltage"=→"Current Bias Voltage [V]":dbl)  [unwired: 2 in]
              n239 = call-dynamic "Supply_Reset.vi"("error in (no error)"=w361, "SupplyControl in"=w349) -> ("error out"=w358:errorcluster, "SupplyControl out"=w357:refnum<class "SupplyControl.lvclass">)  [unwired: 8 in]
              n240 = call-dynamic "Supply_Init.vi"("error in (no error)"=w358, "SupplyControl in"=w357) -> ("error out"=w359:errorcluster, "SupplyControl out"=w356:refnum<class "SupplyControl.lvclass">)  [unwired: 8 in]
              n241 = call-dynamic "Supply_Arm.vi"("error in (no error)"=w359, "SupplyControl in"=w356) -> ("error out"=w372:errorcluster)  [unwired: 8 in, 1 out]
              n242 = call-dynamic "MatrixSwitch.vi"("error in (no error)"=w372, "Action"=T6."Reset", "Switching in"=w345) -> ("error out"=w351:errorcluster, "Switching out"=w352:refnum<class "Switching.lvclass">)  [unwired: 6 in, 1 out]
              n243 = case shown="False" w354 {
                selector: w354 -> [_ w460]
                tunnel: w352 -> [w402 _]
                tunnel: w351 -> [w401 _]
                tunnel: w348 -> [w400 _]
                tunnel: w347 -> [w399 _]
                tunnel: w346 -> [w398 _]
                tunnel: w344 -> [w397 _]
                tunnel: w343 -> [w396 _]
                frame False {
                  n244 = flat-sequence {
                    tunnel: w402 -> [w408]
                    tunnel: [w408] -> w395
                    tunnel: w401 -> [w411]
                    tunnel: w400 -> [w407]
                    tunnel: [w407] -> w394
                    tunnel: w399 -> [w409]
                    tunnel: w398 -> [w406]
                    tunnel: [w406] -> w393
                    tunnel: w397 -> [w405]
                    tunnel: [w405] -> w392
                    tunnel: w396 -> [w404]
                    tunnel: [w404] -> w391
                    tunnel: [w410] -> w390
                    tunnel: w395 -> [w415]
                    tunnel: [w415] -> w378
                    tunnel: w394 -> [w421]
                    tunnel: [w421] -> w377
                    tunnel: w393 -> [w416]
                    tunnel: [w416] -> w376
                    tunnel: w392 -> [w414]
                    tunnel: [w414] -> w375
                    tunnel: w391 -> [w413]
                    tunnel: [w413] -> w374
                    tunnel: w390 -> [w418]
                    tunnel: [w422] -> w373
                    tunnel: w378 -> [w426]
                    tunnel: [w426] -> w389
                    tunnel: w377 -> [w424]
                    tunnel: [w424] -> w388
                    tunnel: w376 -> [w423]
                    tunnel: [w423] -> w387
                    tunnel: w375 -> [w427]
                    tunnel: [w427] -> w386
                    tunnel: w374 -> [w428]
                    tunnel: [w428] -> w385
                    tunnel: w373 -> [w429]
                    tunnel: [w430] -> w384
                    tunnel: w389 -> [w438]
                    tunnel: [w438] -> w383
                    tunnel: w388 -> [w440]
                    tunnel: w387 -> [w437]
                    tunnel: [w437] -> w382
                    tunnel: w386 -> [w436]
                    tunnel: [w436] -> w381
                    tunnel: w385 -> [w435]
                    tunnel: [w435] -> w380
                    tunnel: w384 -> [w441]
                    tunnel: [w439] -> w379
                    tunnel: w383 -> [w447]
                    tunnel: w382 -> [w448]
                    tunnel: w381 -> [w443]
                    tunnel: w380 -> [w442]
                    tunnel: w379 -> [w446]
                    frame #0 {
                      n245 = call-dynamic "Prober_ChuckUpDown.vi"("error in (no error)"=w411, "Direction"=enum16{"up", "down"}."down", "ProbeStationControl in"=w409) -> ("error out"=w410:errorcluster)  [unwired: 6 in, 2 out]
                    }
                    frame #1 {
                      n246 = local write "Status:"("Trimming LCR ..." ("STATUS 1")) -> ()
                      n247 = call-dynamic "Supply_ZeroCheck.vi"("error in (no error)"=w418, "enable/disable"=TRUE, "SupplyControl in"=w416) -> ("error out"=w417:errorcluster)  [unwired: 7 in, 1 out]
                      n248 = call-dynamic "LCR_Init.vi"("error in (no error)"=w417, "LCRControl in"=w421) -> ("error out"=w422:errorcluster)  [unwired: 8 in, 1 out]
                    }
                    frame #2 {
                      n249 = Wait (ms)(milliseconds to wait=1000) -> ()  [unwired: 1 out]
                      n250 = call-dynamic "MuxCardSwitch.vi"("Single Needle"=w428, "Probe Card Channels"=w427, "error in (no error)"=w429, "Switch to channel"=1, "Switching in"=w426) -> ("error out"=w431:errorcluster, "Switching out"=w425:refnum<class "Switching.lvclass">)  [unwired: 4 in, 1 out]
                      n251 = call-dynamic "MatrixSwitch.vi"("error in (no error)"=w431, "Action"=T6."Striptest LCR", "Switching in"=w425) -> ("error out"=w430:errorcluster)  [unwired: 6 in, 2 out]
                    }
                    frame #3 {
                      n252 = call-dynamic "LCR_TrimOC.vi"("error in (no error)"=w441, "LCRControl in"=w440) -> ("error out"=w439:errorcluster)  [unwired: 8 in, 1 out]
                    }
                    frame #4 {
                      w454 = u16 0 items=["Open", "Close"] ("Switch action")
                      n253 = call-dynamic "Supply_ZeroCheck.vi"("error in (no error)"=w446, "enable/disable"=TRUE, "SupplyControl in"=w448) -> ("error out"=w445:errorcluster)  [unwired: 7 in, 1 out]
                      n254 = call-dynamic "MatrixSwitchSingle.vi"("Switch action"=w454, "error in (no error)"=w445, "Matrix Y"=1, "Matrix X"=3, "Switching in"=w447) -> ("error out"=w450:errorcluster, "Switching out"=w451:refnum<class "Switching.lvclass">)  [unwired: 4 in, 1 out]
                      n255 = call-dynamic "MatrixSwitchSingle.vi"("Switch action"=w454, "error in (no error)"=w450, "Matrix Y"=2, "Matrix X"=4, "Switching in"=w451) -> ("error out"=w449:errorcluster, "Switching out"=w444:refnum<class "Switching.lvclass">)  [unwired: 4 in, 1 out]
                      n256 = call-dynamic "MuxCardSwitch.vi"("Single Needle"=w442, "Probe Card Channels"=w443, "error in (no error)"=w449, "Switch to channel"=-1, "Switching in"=w444) -> ()  [unwired: 4 in, 3 out]
                    }
                  }
                  n257 = local write "Bias On/Off:"(TRUE ("Bias On?")) -> ()
                }
                frame True {
                  n258 = property on="Bias On/Off:" class="Bool (strict)"("Blinking"=w460) -> ()  [unwired: 2 in, 2 out]
                  n259 = local write "Status:"("Compliance exceeded\nRUN ABORTED") -> ()
                }
              }
            }
            frame True {
            }
          }
        }
        frame #3 {
          n260 = property on="Bias On/Off:" class="Bool (strict)"() -> ("Blinking"=w462:bool)  [unwired: 2 in, 2 out]
          n261 = case shown="False" w462 {
            tunnel: w463 -> [w467 _]
            tunnel: w461 -> [w464 _]
            frame False {
              w468 = 0
              n262 = property on="Abort" class="Bool (strict)"("DisabledEnum"=w468) -> ()  [unwired: 2 in, 2 out]
              n263 = property on="Auto ReCheck" class="Bool (strict)"("DisabledEnum"=w468) -> ()  [unwired: 2 in, 2 out]
              n264 = local read "Single Needle"() -> (w466:bool)
              n265 = Or(x=w466, y=w467) -> (x .or. y?=w465:bool)
              n266 = case shown="False" w465 {
                tunnel: [w471 FALSE] -> w469
                tunnel: w464 -> [w470 _]
                frame False {
                  n267 = stacked-sequence {
                    tunnel: [_ w480] -> w471
                    tunnel: w470 -> [_ _]
                    frame #0 {
                      n268 = global read "QC_MeasurementSetup.vi" "Striptest Measurement Parameters"() -> (w472:T8)
                      n269 = local write "Status:"("Reference measurement") -> ()
                      n270 = Unbundle By Name(w472) -> ("Measurement switch"=w473:refnum<class "Switching.lvclass">)
                      n271 = call-dynamic "MatrixSwitch.vi"("Action"=T6."Striptest SMU", "Switching in"=w473) -> ()  [unwired: 7 in, 3 out]
                    }
                    frame #1 {
                      n272 = local read "settling\ndelay [ms]"() -> (w479:i32)
                      n273 = call "CurrentCorrection.vi"("Action"=T7."Reference measurement", "settling\ndelay"=w479) -> ("Compliance exceeded?"=w480:bool, "Current Reference 100V"=→"Current Reference 100V":dbl[], "Current Reference 10V"=→"Current Reference 10V":dbl[])  [unwired: 3 in, 2 out]
                    }
                  }
                }
                frame True {
                }
              }
              n274 = case shown="False" w469 {
                frame False {
                  n275 = local write "Status:"("RUN IN PROGRESS" ("STATUS 1")) -> ()
                }
                frame True {
                  n276 = property on="Bias On/Off:" class="Bool (strict)"("Blinking"=TRUE ("Compliance?")) -> ()  [unwired: 2 in, 2 out]
                  n277 = local write "Status:"("Compliance exceeded\nRUN ABORTED") -> ()
                }
              }
            }
            frame True {
            }
          }
        }
        frame #4 {
          n278 = property on="Bias On/Off:" class="Bool (strict)"() -> ("Blinking"=w488:bool)  [unwired: 2 in, 2 out]
          n279 = case shown="False" w488 {
            tunnel: w489 -> [w500 _]
            tunnel: w487 -> [w499 _]
            tunnel: w486 -> [w498 _]
            tunnel: w485 -> [w490 _]
            frame False {
              n280 = Array Size(array=w500) -> (size(s)=w501:i32)
              n281 = local read "Temperature Progression"() -> (w492:T3)
              n282 = local read "probe points per region"() -> (w493:i32[])
              n283 = local read "max scale array"() -> (w496:i32[])
              n284 = local read "min scale array"() -> (w495:i32[])
              n285 = for {
                N: w501 -> [_]
                tunnel: w500 -> [w515] mode=indexing
                tunnel: w499 -> [w514] mode=indexing
                tunnel: w498 -> [w513]
                shift-right: [w507] -> _
                shift-left: 0 -> [w512]
                tunnel: w496 -> [w510] mode=indexing
                tunnel: w495 -> [w511] mode=indexing
                shift-right: [w506] -> _
                shift-left: 0 -> [w508]
                tunnel: w493 -> [w505] mode=indexing
                shift-right: [w503] -> w491
                shift-left: w492 -> [w504]
                tunnel: w490 -> [w502]
                i -> [w509]
                n286 = case shown="True" w515 {
                  tunnel: w514 -> [_ w532]
                  tunnel: w513 -> [_ _]
                  tunnel: w512 -> [w517 w533]
                  tunnel: w511 -> [_ w528]
                  tunnel: w510 -> [_ w525]
                  tunnel: w509 -> [_ w530]
                  tunnel: w508 -> [w519 w527]
                  tunnel: [w516 w526] -> w507
                  tunnel: [w519 w524] -> w506
                  tunnel: w505 -> [_ w523]
                  tunnel: w504 -> [w518 w522]
                  tunnel: [w518 w521] -> w503
                  tunnel: w502 -> [_ w520]
                  frame False {
                    n287 = Increment(x=w517) -> (x+1=w516:i32)
                  }
                  frame True {
                    n288 = local write "Show:"(w533) -> ()
                    n289 = Unbundle By Name(w532) -> ("Region"=→"Probing Region:":string, "ProbePoints"=w529:T14)
                    n290 = while {
                      tunnel: w530 -> [w535]
                      tunnel: w529 -> [w555]
                      shift-right: [w548] -> _
                      shift-left: w528 -> [w537]
                      shift-right: [w549] -> w524
                      shift-left: w527 -> [w550]
                      tunnel: w525 -> [w547]
                      tunnel: w523 -> [_]
                      shift-right: [w545] -> w521
                      shift-left: w522 -> [w546]
                      tunnel: w520 -> [w534]
                      i -> [w551]
                      stop <- w554 stop-if-true
                      n291 = Index Array(array=w555, index=w537) -> (element=w556:T15)
                      n292 = Equal To 0?(x=w550) -> (x = 0?=w557:bool)
                      n293 = Equal?(x=w537, y=w547) -> (x = y?=w536:bool)
                      n294 = case shown="True" w557 {
                        frame False {
                        }
                        frame True {
                          n295 = local read "Probe Card Channels"() -> (w1105:i32)
                          n296 = local read "total strip number"() -> (w1106:u32)
                          n297 = Divide(x=w1106, y=w1105) -> (x/y=w1104:dbl)
                          n298 = To Long Integer(number=w1104) -> (32bit integer=w1103:i32)
                          n299 = call "RunTime.vi"("no. measurements"=w1103, "Flag"=1) -> ()  [unwired: 2 in, 4 out]
                        }
                      }
                      n300 = case shown="True" w536 {
                        tunnel: w535 -> [_ w558]
                        frame False {
                        }
                        frame True {
                          n301 = stacked-sequence {
                            tunnel: w558 -> [_ w562 w567]
                            frame #0 {
                              n302 = Wait (ms)(milliseconds to wait=100) -> ()  [unwired: 1 out]
                            }
                            frame #1 {
                              n303 = Increment(x=w562) -> (x+1=w565:i32)
                              n304 = Multiply(x=w565, y=111) -> (x*y=w563:i32)
                              n305 = Current VI's Path() -> (path=w560:path)
                              n306 = call "SaveJPEG.vi"("Picture No."=w563, "Test"="Striptest", "File Path Control"=w560) -> ()  [unwired: 2 out]
                            }
                            frame #2 {
                              n307 = local read "probe points per region"() -> (w569:i32[])
                              n308 = Index Array(array=w569, index=w567) -> ()  [unwired: 1 out]
                              n309 = local read "Probing Region:"() -> (w566:string)
                              n310 = call "SaveStriptestRecoveryFiles.vi"("Array Titles"="ProbeplanIndex Current[nA] Capacitance[pF] Resistance[MOhm]", "Strip Segment"=w566, "Region #"=w567) -> ()  [unwired: 3 in, 2 out]
                            }
                          }
                        }
                      }
                      n311 = Unbundle By Name(w556) -> ("CardViable?"=w542:bool)
                      n312 = property on="Bias On/Off:" class="Bool (strict)"() -> ("Blinking"=w552:bool)  [unwired: 2 in, 2 out]
                      n313 = property on="Bias On/Off:" class="Bool (strict)"() -> ("Blinking"=w544:bool)  [unwired: 2 in, 2 out]
                      n314 = local read "Abort"() -> (w540:bool)
                      n315 = Not(x=w544) -> (.not. x?=w543:bool)
                      n316 = Not(x=w540) -> (.not. x?=w539:bool)
                      n317 = Compound Arithmetic op=AND(w542, w543, w539) -> (w541:bool)
                      n318 = Build Array(w552, "Abort", w536) -> (w553:bool[])
                      n319 = Or Array Elements(Boolean array=w553) -> (logical OR=w554:bool)
                      n320 = case shown="True" w541 {
                        tunnel: w535 -> [_ w588]
                        tunnel: w555 -> [_ w587]
                        tunnel: w537 -> [w570 w582]
                        tunnel: w551 -> [_ w586]
                        tunnel: w550 -> [w573 w585]
                        tunnel: [w573 w584] -> w549
                        tunnel: [w571 w583] -> w548
                        tunnel: w546 -> [w572 w581]
                        tunnel: [w572 w580] -> w545
                        tunnel: w534 -> [_ w574]
                        frame False {
                          n321 = Increment(x=w570) -> (x+1=w571:i32)
                        }
                        frame True {
                          n322 = global read "QC_MeasurementSetup.vi" "Striptest Measurement Parameters"() -> (w578:T8)
                          n323 = Unbundle By Name(w578) -> ("ProbeStation"=w577:refnum<class "ProbeStationControl.lvclass">, "Measurement switch"=w579:refnum<class "Switching.lvclass">, "Temperature Readout"=w575:enum16{"Read Arduino", "Enter manually"}, "Arduino"=w576:refnum<class "ArduinoControl.lvclass">)
                          n324 = stacked-sequence {
                            tunnel: w588 -> [w602 w883 w971 w1069 _]
                            tunnel: w587 -> [w593 _ _ _ _]
                            tunnel: w582 -> [w592 _ _ _ w1087]
                            tunnel: w585 -> [_ _ _ _ w1096]
                            tunnel: w586 -> [_ w882 w970 w1068 w1085]
                            tunnel: [_ _ _ _ w1088] -> w584
                            tunnel: [_ _ _ _ w1095] -> w583
                            tunnel: w581 -> [_ w878 _ _ _]
                            tunnel: [_ w877 _ _ _] -> w580
                            tunnel: w579 -> [_ w881 w969 _ _]
                            tunnel: w577 -> [w591 _ _ _ _]
                            tunnel: w576 -> [_ w880 _ _ _]
                            tunnel: w575 -> [_ w879 _ _ _]
                            tunnel: w574 -> [w589 w876 w968 _ _]
                            frame #0 {
                              # "If probepoint label defined as Strip or Channel, use\nthat as the channel number in the data array."
                              n325 = local read "Abort"() -> (w598:bool)
                              n326 = Index Array(array=w593, index=w592) -> (element=w609:T15)
                              n327 = local write "disabled channels"(i32[] []) -> ()
                              n328 = Or(x=w598, y=w589) -> (x .or. y?=w597:bool)
                              n329 = Unbundle(w609) -> ("Label"=w605:string)  [unwired: 3 out]
                              "Probe Point:" <- w605
                              n330 = Format Into String(format string="Moving to %s", w605) -> (resulting string=w608:string)  [unwired: 2 in, 1 out]
                              n331 = local write "Status:"(w608) -> ()
                              n332 = local read "Probe Card Channels"() -> (w599:i32)
                              n333 = case shown="False" w597 {
                                tunnel: w602 -> [w868 _]
                                tunnel: w592 -> [w869 _]
                                tunnel: w599 -> [w870 _]
                                tunnel: w591 -> [w866 _]
                                frame False {
                                # "Move to Strip"
                                n334 = local read "Single Needle"() -> (w872:bool)
                                n335 = call "MoveToStrip.vi"("Single Needle"=w872, "Strip No."=w869, "Region"=w868, "ProbeStationControl in"=w866) -> ("Z [µm]"=w867:i32)  [unwired: 5 in, 2 out]
                                n336 = Initialize Array(w867, w870, 1) -> (w873:i32[][])
                                n337 = local read "Z profile"() -> (w875:i32[][])
                                n338 = Replace Array Subset(array=w875, new element=w873, index (row)=w869, index (col)=w868) -> (w874:i32[][])
                                n339 = local write "Z profile"(w874) -> ()
                                }
                                frame True {
                                }
                              }
                              n340 = xnode "Match Regular Expression"("input string"=w605, "regular expression"="(Strip|Channel)\\s+(\\d+)", "ignore case? (F)"=TRUE) -> ("submatch 2"=w596:string)  [unwired: 3 in, 6 out]
                              n341 = Empty String/Path?(string/path=w596) -> (empty?=w595:bool)
                              n342 = Not(x=w595) -> (.not. x?=w594:bool)
                              n343 = case shown="True" w594 {
                                tunnel: [w611 w621] -> w603
                                tunnel: w592 -> [w613 w619]
                                tunnel: w599 -> [w612 w620]
                                tunnel: w593 -> [_ w618]
                                frame False {
                                n344 = for {
                                N: w612 -> [_]
                                tunnel: w613 -> [w616]
                                tunnel: [w614] -> w611 mode=indexing
                                i -> [w617]
                                # "Actually use the probepoint\nindex"
                                n345 = Add(x=w616, y=w617) -> (x+y=w615:i32)
                                n346 = Increment(x=w615) -> (x+1=w614:i32)
                                }
                                }
                                frame True {
                                n347 = for {
                                N: w620 -> [_]
                                tunnel: [w630] -> w621 mode=indexing
                                tunnel: w619 -> [w627]
                                tunnel: w618 -> [w625]
                                i -> [w628]
                                n348 = Add(x=w627, y=w628) -> (x+y=w626:i32)
                                n349 = Index Array(array=w625, index=w626) -> (element=w624:T15)
                                n350 = Unbundle By Name(w624) -> ("Label"=w623:string)
                                n351 = xnode "Match Regular Expression"("input string"=w623, "regular expression"="(Strip|Channel)\\s+(\\d+)") -> ("submatch 2"=w622:string)  [unwired: 4 in, 6 out]
                                n352 = Scan From String(format string="%d", input string=w622) -> (output 1=w630:i32)  [unwired: 3 in, 3 out]
                                }
                                }
                              }
                              n353 = To Double Precision Float(number=w603) -> (double precision float=w600:dbl[])
                              n354 = call "MultiRegionData.vi"("Action"=T5."Add Array", "Array No."=0 ("Array Size / Index"), "Array IN"=w600, "Region index"=w602) -> ()  [unwired: 2 in, 2 out]
                            }
                            frame #1 {
                              # "Pinholes"
                              n355 = stacked-sequence {
                                tunnel: w876 -> [w899 w920]
                                tunnel: w883 -> [_ w922]
                                tunnel: w882 -> [_ w921]
                                tunnel: w881 -> [w898 _]
                                tunnel: w880 -> [w896 _]
                                tunnel: w879 -> [w897 _]
                                tunnel: w878 -> [w890 _]
                                tunnel: [w888 _] -> w877
                                frame #0 {
                                n356 = Unbundle By Name(w890) -> ("Time Array"=w892:string[], "Temperature Array [°C]"=w887:dbl[], "Humidity Array [RH %]"=w886:dbl[])
                                n357 = case shown="\"Read Arduino\", Default" w897 {
                                tunnel: w896 -> [w907 _]
                                tunnel: [w906 _] -> w895
                                tunnel: w887 -> [w902 w911]
                                tunnel: w886 -> [w903 w913]
                                tunnel: [w901 w910] -> w885
                                tunnel: [w900 w909] -> w884
                                frame "Read Arduino", Default {
                                n358 = call "ArduinoRead.vi"("Arduino function"=enum16{"T/RH", "Interlock", "Edgesense"}."T/RH", "ArduinoControl in"=w907) -> ("error out"=w906:errorcluster, "rel. Humidity [%]"=w904:dbl, "Temperature [°C]"=w905:dbl)  [unwired: 4 in, 3 out]
                                n359 = Build Array (concatenate)(w902, w905) -> (w901:dbl[])
                                n360 = Build Array (concatenate)(w903, w904) -> (w900:dbl[])
                                }
                                frame "Enter manually" {
                                n361 = Index Array(array=w911, index=0) -> (element=w912:dbl)
                                n362 = Index Array(array=w913, index=0) -> (element=w914:dbl)
                                n363 = Build Array (concatenate)(w911, w912) -> (w910:dbl[])
                                n364 = Build Array (concatenate)(w913, w914) -> (w909:dbl[])
                                }
                                }
                                n365 = call "RunTime.vi"("Probing done - new estimation"=FALSE, "Flag"=0) -> ("Time so far"=w891:string)  [unwired: 2 in, 3 out]
                                n366 = Build Array (concatenate)(w892, w891) -> (w889:string[])
                                n367 = case shown="False" w899 {
                                tunnel: w898 -> [w919 _]
                                tunnel: w895 -> [w918 _]
                                frame False {
                                n368 = call-dynamic "MatrixSwitch.vi"("error in (no error)"=w918, "Action"=T6."Striptest SMU", "Switching in"=w919) -> ()  [unwired: 6 in, 3 out]
                                }
                                frame True {
                                }
                                }
                                n369 = Bundle By Name(cluster=w890, "Time Array"=w889, "Temperature Array [°C]"=w885, "Humidity Array [RH %]"=w884) -> (w888:T3)
                                }
                                frame #1 {
                                n370 = local read "Abort"() -> (w923:bool)
                                n371 = case shown="False" w923 {
                                tunnel: w922 -> [w931 _]
                                tunnel: w921 -> [_ _]
                                tunnel: w920 -> [w925 _]
                                frame False {
                                w924 = T5."Add Array" ("Action")
                                n372 = case shown="True" w925 {
                                tunnel: [w943 w956] -> w926
                                tunnel: [w940 w955] -> w930
                                frame False {
                                n373 = local read "Thresholds:"() -> (w942:T2)
                                n374 = Unbundle By Name(w942) -> ("Current [nA]"=w941:dbl)
                                n375 = case shown="True" "Rolling\nCurrent Readout" {
                                tunnel: [w948 w950] -> w943
                                tunnel: w941 -> [w944 w953]
                                tunnel: [w947 w952] -> w940
                                tunnel: [w946 w951] -> w939
                                tunnel: "settling\ndelay [ms]" -> [w945 w949]
                                frame False {
                                n376 = call "Pinholes.vi"("Current Threshold [nA]"=w944, "settling\ndelay"=w945) -> ("excluded channels"=w946:i32[], "Current [nA]"=w948:dbl[], "Flag"=w947:i32[])  [unwired: 3 in]
                                }
                                frame True {
                                n377 = call "PinholesRolling.vi"("Current Threshold [nA]"=w953, "settling\ndelay"=w949) -> ("excluded channels"=w951:i32[], "Current [nA]"=w950:dbl[], "Flag"=w952:i32[])  [unwired: 3 in]
                                }
                                }
                                "disabled channels" <- w939
                                }
                                frame True {
                                n378 = local read "Probe Card Channels"() -> (w954:i32)
                                n379 = for {
                                N: w954 -> [_]
                                tunnel: [w958] -> w956 mode=indexing
                                tunnel: [w957] -> w955 mode=indexing
                                # "Simulate"
                                n380 = Random Number (0-1)() -> (number: 0 to 1=w961:dbl)
                                n381 = Greater?(x=w961, y=0.95) -> (0:w962:bool)
                                n382 = case shown="True" w962 {
                                tunnel: [w966 5000.0] -> w958
                                tunnel: w961 -> [w966 _]
                                frame False {
                                }
                                frame True {
                                }
                                }
                                n383 = Greater?(x=w958, y=50.0) -> (0:w959:bool)
                                n384 = case shown="True" w959 {
                                tunnel: [0 1] -> w957
                                frame False {
                                }
                                frame True {
                                }
                                }
                                }
                                }
                                }
                                n385 = Get Date/Time String(want seconds? (F)=TRUE) -> (time string=→"Last Probe at:":string)  [unwired: 2 in, 1 out]
                                n386 = local write "Status:"("Measuring Ipinhole") -> ()
                                n387 = To Double Precision Float(number=w930) -> (double precision float=w929:dbl[])
                                n388 = Index Array(array=w926, index=0) -> (element=→"Current [nA]:":dbl)
                                n389 = call "MultiRegionData.vi"("Action"=w924, "Array No."=1, "Array IN"=w926, "Region index"=w931) -> ()  [unwired: 2 in, 2 out]
                                n390 = call "MultiRegionData.vi"("Action"=w924, "Array No."=2, "Array IN"=w929, "Region index"=w931) -> ()  [unwired: 2 in, 2 out]
                                }
                                frame True {
                                }
                                }
                                }
                              }
                            }
                            frame #2 {
                              # "Capacitance and Resistance"
                              n391 = stacked-sequence {
                                seq-local: [_ _ w984 _] -> [_ _ _ w1046]
                                tunnel: w971 -> [_ _ w991 _]
                                tunnel: w970 -> [_ _ _ _]
                                tunnel: w968 -> [w973 w977 w983 w1045]
                                tunnel: w969 -> [w972 w976 w982 w1044]
                                frame #0 {
                                n392 = case shown="False" w973 {
                                tunnel: w972 -> [w974 _]
                                frame False {
                                n393 = call-dynamic "MatrixSwitch.vi"("Action"=T6."Ground", "Switching in"=w974) -> ()  [unwired: 7 in, 3 out]
                                }
                                frame True {
                                }
                                }
                                }
                                frame #1 {
                                n394 = case shown="False" w977 {
                                tunnel: w976 -> [w979 _]
                                frame False {
                                n395 = call-dynamic "MatrixSwitch.vi"("Action"=T6."Striptest LCR", "Switching in"=w979) -> ()  [unwired: 7 in, 3 out]
                                }
                                frame True {
                                }
                                }
                                n396 = local write "Status:"("Measuring capacitance..." ("STATUS 1")) -> ()
                                }
                                frame #2 {
                                w981 = T5."Add Array" ("Action")
                                w987 = 0
                                n397 = local read "Probe Card Channels"() -> (w984:i32)
                                n398 = local read "disabled channels"() -> (w986:i32[])
                                n399 = for {
                                N: w984 -> [_]
                                tunnel: [w1000] -> w985 mode=indexing
                                tunnel: [w999] -> w988 mode=indexing
                                tunnel: w986 -> [w996]
                                tunnel: w984 -> [w998]
                                tunnel: w983 -> [w995]
                                tunnel: w982 -> [w994]
                                i -> [w997]
                                n400 = case shown="True" w995 {
                                tunnel: [w1009 w1038] -> w1000
                                tunnel: [w1008 w1037] -> w999
                                tunnel: w998 -> [w1005 _]
                                tunnel: w997 -> [w1003 _]
                                tunnel: w996 -> [w1004 _]
                                tunnel: w994 -> [w1001 _]
                                frame False {
                                n401 = Increment(x=w1003) -> (x+1=w1002:i32)
                                n402 = Search 1D Array(1D array=w1004, element=w1002) -> (index of element=w1007:i32)  [unwired: 1 in]
                                n403 = Less Than 0?(x=w1007) -> (x < 0?=w1006:bool)
                                n404 = case shown="True" w1006 {
                                tunnel: [w1012 w1018] -> w1009
                                tunnel: [w1010 w1017] -> w1008
                                tunnel: w1005 -> [_ w1016]
                                tunnel: w1002 -> [_ w1015]
                                tunnel: w1004 -> [_ w1014]
                                tunnel: w1001 -> [_ w1013]
                                frame False {
                                w1012 = -1.0
                                n405 = Divide(x=w1012, y=1000000.0) -> (x/y=w1010:dbl)
                                }
                                frame True {
                                n406 = stacked-sequence {
                                tunnel: w1016 -> [w1021 _ _]
                                tunnel: w1015 -> [w1023 _ _]
                                tunnel: w1014 -> [w1022 _ _]
                                tunnel: [_ _ w1029] -> w1018
                                tunnel: [_ _ w1028] -> w1017
                                tunnel: w1013 -> [w1020 _ _]
                                frame #0 {
                                n407 = local read "Single Needle"() -> (w1019:bool)
                                n408 = call-dynamic "MuxCardSwitch.vi"("Single Needle"=w1019, "Probe Card Channels"=w1021, "disabled channels"=w1022, "Switch to channel"=w1023, "Switching in"=w1020) -> ()  [unwired: 4 in, 3 out]
                                }
                                frame #1 {
                                n409 = local read "settling\ndelay [ms]"() -> (w1024:i32)
                                n410 = Wait (ms)(milliseconds to wait=w1024) -> ()  [unwired: 1 out]
                                }
                                frame #2 {
                                n411 = global read "QC_MeasurementSetup.vi" "Striptest Measurement Parameters"() -> (w1027:T8)
                                n412 = Unbundle By Name(w1027) -> ("LCR"=w1026:refnum<class "LCRControl.lvclass">, "AC frequency [Hz]"=w1025:i32)
                                n413 = call-dynamic "LCR_Readout.vi"(10:w1025, "LCRControl in"=w1026) -> ("Resistance in Ohm"=w1028:dbl, "Capacitance in pF"=w1029:dbl)  [unwired: 6 in, 2 out]
                                }
                                }
                                }
                                }
                                }
                                frame True {
                                n414 = Random Number (0-1)() -> (number: 0 to 1=w1040:dbl)
                                n415 = Random Number (0-1)() -> (number: 0 to 1=w1043:dbl)
                                n416 = Multiply(x=w1043, y=34.0) -> (x*y=w1031:dbl)
                                n417 = Multiply(x=w1040, y=1.2) -> (x*y=w1035:dbl)
                                n418 = Subtract(x=w1031, y=17.0) -> (x-y=w1030:dbl)
                                n419 = Subtract(x=w1035, y=0.6) -> (x-y=w1034:dbl)
                                n420 = Add(x=w1030, y=64.0) -> (x+y=w1038:dbl)
                                n421 = Add(x=1.5 ("Resistance"), y=w1034) -> (x+y=w1037:dbl)
                                }
                                }
                                }
                                n422 = Index Array(array=w985, index=w987) -> (element=→"Capacitance [pF]:":dbl)
                                n423 = Index Array(array=w988, index=w987) -> (element=→"Reistance [MW]:":dbl)
                                n424 = call "MultiRegionData.vi"("Action"=w981, "Array No."=3, "Array IN"=w985, "Region index"=w991) -> ()  [unwired: 2 in, 2 out]
                                n425 = call "MultiRegionData.vi"("Action"=w981, "Array No."=4, "Array IN"=w988, "Region index"=w991) -> ()  [unwired: 2 in, 2 out]
                                }
                                frame #3 {
                                n426 = case shown="False" w1045 {
                                tunnel: w1046 -> [w1049 _]
                                tunnel: w1044 -> [w1047 _]
                                frame False {
                                n427 = local read "Single Needle"() -> (w1048:bool)
                                n428 = call-dynamic "MuxCardSwitch.vi"("Single Needle"=w1048, "Probe Card Channels"=w1049, "Switch to channel"=-1, "Switching in"=w1047) -> ()  [unwired: 5 in, 3 out]
                                }
                                frame True {
                                }
                                }
                                }
                              }
                            }
                            frame #3 {
                              # "If selected region is CURRENT region being probed,\nuse number probed so far\notherwise total number of probepoints in this region"
                              n429 = local read "Region Indices"() -> (w1071:i32[])
                              n430 = Index Array(array=w1071, index="Show:") -> (element=w1067:i32)
                              n431 = Equal?(x=w1067, y=w1069) -> (x = y?=w1070:bool)
                              n432 = case shown="True" w1070 {
                                tunnel: w1068 -> [_ w1083]
                                tunnel: [w1079 w1082] -> w1066
                                tunnel: w1067 -> [w1078 _]
                                frame False {
                                n433 = local read "probe points per region"() -> (w1080:i32[])
                                n434 = Index Array(array=w1080, index=w1078) -> (element=w1079:i32)
                                }
                                frame True {
                                n435 = local read "Probe Card Channels"() -> (w1081:i32)
                                n436 = Add(x=w1081, y=w1083) -> (x+y=w1082:i32)
                                }
                              }
                              n437 = global read "ProbePlanParams.vi" "ProbePlan Parameters IN"() -> (w1052:T11)
                              n438 = Unbundle By Name(w1052) -> ("Test ProbePoints.Strip length [cm]"=w1051:dbl[])
                              n439 = local read "max scale array"() -> (w1063:i32[])
                              n440 = local read "min scale array"() -> (w1065:i32[])
                              n441 = local read "Thresholds:"() -> (w1077:T2)
                              n442 = Index Array(array=w1063, index="Show:") -> (element=w1060:i32)
                              n443 = Index Array(array=w1065, index="Show:") -> (element=w1062:i32)
                              n444 = call "DisplayStriptestData.vi"("Strip Lengths [cm]"=w1051, "min scale array"=w1065, "max scale array"=w1063, "# probed"=w1066, "Display Stats?"=TRUE, "Thresholds:"=w1077, "Region"=w1067) -> ("Defects"=→"Defects":i32[][], "Resistance [MW]"=→"Resistance [MW]":cluster{u32, i32, "Array OUT":dbl[]}, "Capacitance [pF]"=→"Capacitance [pF]":cluster{u32, i32, "Array OUT":dbl[]}, "Current [nA]"=→"Current [nA]":cluster{u32, i32, "Array OUT":dbl[]}, "Strip Quality Data"=w1073:T16)
                              n445 = Increment(x=w1060) -> (x+1=w1059:i32)
                              n446 = Increment(x=w1062) -> (x+1=w1061:i32)
                              n447 = property on="Capacitance [pF]" class="WFGraph (strict)"("XScale.Minimum"=w1061) -> ()  [unwired: 2 in, 2 out]
                              n448 = property on="Resistance [MW]" class="WFGraph (strict)"("XScale.Minimum"=w1061) -> ()  [unwired: 2 in, 2 out]
                              n449 = property on="Current [nA]" class="WFGraph (strict)"("XScale.Minimum"=w1061) -> ()  [unwired: 2 in, 2 out]
                              n450 = property on="Defects" class="IntGraph (strict)"("XScale.Minimum"=w1061) -> ()  [unwired: 2 in, 2 out]
                              n451 = property on="Capacitance [pF]" class="WFGraph (strict)"("XScale.Maximum"=w1059) -> ()  [unwired: 2 in, 2 out]
                              n452 = Increment(x=w1059) -> (x+1=w1058:i32)
                              n453 = property on="Resistance [MW]" class="WFGraph (strict)"("XScale.Maximum"=w1059) -> ()  [unwired: 2 in, 2 out]
                              n454 = property on="Current [nA]" class="WFGraph (strict)"("XScale.Maximum"=w1059) -> ()  [unwired: 2 in, 2 out]
                              n455 = property on="Defects" class="IntGraph (strict)"("XScale.Maximum"=w1058) -> ()  [unwired: 2 in, 2 out]
                              n456 = Unbundle By Name(w1073) -> ("pass Rate in %"=→"% OK:":dbl, "Bad channel list"=→"Bad Strip List":i32[], "No of bad strips"=w1056:i32, "Number of defects per category"=→"defect type array":i32[])
                              n457 = local write "# total defects:"(w1056) -> ()
                            }
                            frame #4 {
                              n458 = Increment(x=w1087) -> (x+1=w1095:i32)
                              n459 = call "RunTime.vi"("Probing done - new estimation"=TRUE, "Flag"=0) -> ("Estimated Completion Time"=w1092:string, "Time so far"=→"Run Duration:":string)  [unwired: 2 in, 2 out]
                              n460 = Scan From String(format string="%s %s", input string=w1092) -> (output 2=→"Estimated Completion:":string)  [unwired: 5 in, 3 out]
                              n461 = local read "Probe Card Channels"() -> (w1086:i32)
                              n462 = Add(x=w1086, y=w1096) -> (x+y=w1088:i32)
                              n463 = case shown="True" FALSE {
                                tunnel: w1086 -> [_ w1102]
                                tunnel: w1085 -> [_ w1101]
                                frame False {
                                }
                                frame True {
                                # "save image if required"
                                n464 = Quotient & Remainder(x=w1101, y=w1102) -> (floor(x/y)=w1100:i32)  [unwired: 1 out]
                                n465 = Increment(x=w1100) -> (x+1=w1099:i32)
                                n466 = Current VI's Path() -> (path=w1097:path)
                                n467 = call "SaveJPEG.vi"("Picture No."=w1099, "Test"="Striptest", "File Path Control"=w1097) -> ()  [unwired: 2 out]
                                }
                              }
                              n468 = local write "# probed"(w1088) -> ()
                            }
                          }
                        }
                      }
                    }
                    n469 = Increment(x=w533) -> (x+1=w526:i32)
                  }
                }
              }
              n470 = local write "Temperature Progression"(w491) -> ()
            }
            frame True {
            }
          }
        }
        frame #5 {
          # "Ramp down volts now"
          n471 = flat-sequence {
            tunnel: w1108 -> [w1128]
            tunnel: w1109 -> [w1127]
            frame #0 {
              n472 = case shown="False" w1128 {
                tunnel: w1127 -> [w1130 _]
                frame False {
                  w1135 = "0"
                  n473 = call-dynamic "Prober_ChuckUpDown.vi"("Direction"=enum16{"up", "down"}."down", "ProbeStationControl in"=w1130) -> ("error out"=w1132:errorcluster, "ProbeStationControl out"=w1131:refnum<class "ProbeStationControl.lvclass">)  [unwired: 7 in, 1 out]
                  n474 = call-dynamic "Prober_MoveToXYZTheta.vi"("Theta location [mdeg]"="none", "ProbeStationControl in"=w1131, "error in (no error)"=w1132, "Z location [µm]"="down", "Y location [µm]"=w1135, "X location [µm]"=w1135) -> ()  [unwired: 3 in, 3 out]
                }
                frame True {
                }
              }
            }
            frame #1 {
              n475 = property on="Abort" class="Bool (strict)"("DisabledEnum"=2) -> ()  [unwired: 2 in, 2 out]
              n476 = local read "# probed"() -> (w1139:i32)
              n477 = Current VI's Path() -> (path=w1136:path)
              n478 = call "SaveJPEG.vi"("Picture No."=w1139, "Test"="Striptest", "File Path Control"=w1136) -> ()  [unwired: 2 out]
            }
          }
          n479 = property on="Bias On/Off:" class="Bool (strict)"() -> ("Blinking"=w1120:bool)  [unwired: 2 in, 2 out]
          n480 = local read "Abort"() -> (w1121:bool)
          n481 = Not Or(1:w1121, 2:w1120) -> (0:w1119:bool)
          n482 = Build Array(w1119, w1120, w1121) -> (w1122:bool[])
          n483 = Search 1D Array(1D array=w1122, element=TRUE) -> (index of element=w1124:i32)  [unwired: 1 in]
          n484 = Increment(x=w1124) -> (x+1=w1110:i32)
          n485 = global read "QC_RunInformation.vi" "Run info"() -> (w1113:T10)
          n486 = Pick Line(multi-line string=" null\n Run ended normally.\n Compliance exceeded. \n Run aborted early.", line index=w1110) -> (output string=w1111:string)  [unwired: 1 in]
          n487 = Bundle By Name(cluster=w1113, "End of Run comment:"=w1111) -> (w1112:T10)
          n488 = global write "QC_RunInformation.vi" "Run info"(w1112) -> ()
          n489 = Concatenate Strings(" End of Run.", "\r\n", w1111) -> (w1114:string)
          n490 = Concatenate Strings(w1111, "\r\n", "RAMPING DOWN VOLTS") -> (w1117:string)
          n491 = stacked-sequence {
            tunnel: w1117 -> [w1140 _ _ _]
            tunnel: w1114 -> [_ _ w1144 _]
            tunnel: w1108 -> [_ w1141 _ _]
            frame #0 {
              n492 = local write "Status:"(w1140) -> ()
            }
            frame #1 {
              n493 = case shown="False" w1141 {
                frame False {
                  n494 = global read "QC_MeasurementSetup.vi" "Striptest Measurement Parameters"() -> (w1143:T8)
                  n495 = Unbundle By Name(w1143) -> ("SMU"=w1142:refnum<class "SupplyControl.lvclass">)
                  n496 = call-dynamic "Supply_Stby.vi"("SupplyControl in"=w1142) -> ()  [unwired: 9 in, 2 out]
                }
                frame True {
                }
              }
            }
            frame #2 {
              n497 = local write "Status:"(w1144) -> ()
            }
            frame #3 {
              w1147 = 0
              n498 = property on="Save Data" class="Bool (strict)"("DisabledEnum"=w1147) -> ()  [unwired: 2 in, 2 out]
              n499 = property on="Quit w/o saving" class="Bool (strict)"("DisabledEnum"=w1147) -> ()  [unwired: 2 in, 2 out]
              n500 = property on="ReCheck" class="Bool"("DisabledEnum"=w1147) -> ()  [unwired: 2 in, 2 out]
              n501 = property on="Auto ReCheck" class="Bool (strict)"("DisabledEnum"=1) -> ()  [unwired: 2 in, 2 out]
              n502 = local write "Status:"("Run finished. \nSave data?" ("STATUS 1")) -> ()
            }
          }
        }
        frame #6 {
          w1159 = ""
          n503 = stacked-sequence {
            tunnel: [w1181 _ _ _] -> w1177
            tunnel: [w1180 _ _ _] -> w1176
            tunnel: w1170 -> [_ w1290 w1306 _]
            tunnel: w1169 -> [w1179 _ _ _]
            frame #0 {
              # "Loop and await decision on whether to save or junk data"
              n504 = local read "Show:"() -> (w1182:u16)
              n505 = while {
                shift-right: [w1190] -> _
                shift-left: w1182 -> [w1191]
                tunnel: ["Save Data"] -> w1180
                tunnel: ["Quit w/o saving"] -> w1181
                tunnel: w1179 -> [w1183]
                stop <- w1194 stop-if-true
                # "display data if selected region changes"
                n506 = Wait (ms)(milliseconds to wait=u32 200) -> ()  [unwired: 1 out]
                n507 = local read "Show:"() -> (w1192:u16)
                n508 = Not Equal?(x=w1192, y=w1191) -> (x != y?=w1193:bool)
                n509 = Or(x="ReCheck", y="Auto ReCheck") -> (x .or. y?=w1185:bool)
                n510 = case shown="True" w1185 {
                  tunnel: "Auto ReCheck" -> [_ w1196]
                  tunnel: w1183 -> [_ w1195]
                  frame False {
                  }
                  frame True {
                    n511 = case shown="True" w1196 {
                      tunnel: w1195 -> [_ w1228]
                      frame False {
                        n512 = local read "probe points per region"() -> (w1203:i32[])
                        n513 = local read "Region Indices"() -> (w1204:i32[])
                        n514 = local read "Show:"() -> (w1202:u16)
                        n515 = Index Array(array=w1204, index=w1202) -> (element=w1201:i32)
                        n516 = Index Array(array=w1203, index=w1202) -> (element=w1200:i32)
                        n517 = flat-sequence {
                          tunnel: w1201 -> [w1205]
                          tunnel: w1200 -> [w1209]
                          tunnel: [w1205] -> w1199
                          tunnel: [w1209] -> w1198
                          tunnel: [w1208] -> w1197
                          tunnel: w1199 -> [w1227]
                          tunnel: w1198 -> [w1224]
                          tunnel: w1197 -> [w1213]
                          frame #0 {
                            n518 = local read "Probe Card Channels"() -> (w1206:i32)
                            n519 = local read "Auto ReCheck"() -> (w1207:bool)
                            n520 = local read "Thresholds:"() -> (w1210:T2)
                            n521 = call "ReCheckStrips.vi"("Probe Card Channels"=w1206, "Auto Re-Check"=w1207, "Thresholds"=w1210, "region in"=w1205, "Number of strips probed"=w1209) -> ("Thresholds copy"=w1208:T17)  [unwired: 6 in]
                            n522 = local write "Thresholds:"(w1208) -> ()
                          }
                          frame #1 {
                            n523 = global read "ProbePlanParams.vi" "ProbePlan Parameters IN"() -> (w1212:T11)
                            n524 = Unbundle By Name(w1212) -> ("Test ProbePoints.Strip length [cm]"=w1211:dbl[])
                            n525 = local read "max scale array"() -> (w1226:i32[])
                            n526 = local read "min scale array"() -> (w1225:i32[])
                            n527 = call "DisplayStriptestData.vi"("Strip Lengths [cm]"=w1211, "min scale array"=w1225, "max scale array"=w1226, "# probed"=w1224, "Display Stats?"=TRUE, "Thresholds:"=w1213, "Region"=w1227) -> ("Defects"=w1219:i32[][], "Resistance [MW]"=w1220:cluster{u32, i32, "Array OUT":dbl[]}, "Capacitance [pF]"=w1222:cluster{u32, i32, "Array OUT":dbl[]}, "Current [nA]"=w1221:cluster{u32, i32, "Array OUT":dbl[]}, "Strip Quality Data"=w1218:T16)
                            n528 = local write "Defects"(w1219) -> ()
                            n529 = local write "Current [nA]"(w1221) -> ()
                            n530 = local write "Capacitance [pF]"(w1222) -> ()
                            n531 = local write "Resistance [MW]"(w1220) -> ()
                            n532 = Unbundle By Name(w1218) -> ("pass Rate in %"=w1217:dbl, "Bad channel list"=w1216:i32[], "No of bad strips"=w1215:i32, "Defect description list"=w1214:i32[])
                            n533 = local write "% OK:"(w1217) -> ()
                            n534 = local write "Bad Strip List"(w1216) -> ()
                            n535 = local write "# total defects:"(w1215) -> ()
                            n536 = local write "defect type array"(w1214) -> ()
                          }
                        }
                      }
                      frame True {
                        n537 = flat-sequence {
                          tunnel: w1228 -> [w1229]
                          frame #0 {
                            n538 = local read "Region Indices"() -> (w1230:i32[])
                            n539 = Array Size(array=w1230) -> (size(s)=w1231:i32)
                            n540 = for {
                              N: w1231 -> [_]
                              tunnel: w1230 -> [w1233] mode=indexing
                              tunnel: w1229 -> [w1232] mode=indexing
                              n541 = case shown="True" w1232 {
                                tunnel: w1233 -> [_ w1237]
                                frame False {
                                }
                                frame True {
                                n542 = local read "probe points per region"() -> (w1239:i32[])
                                n543 = Index Array(array=w1239, index=w1237) -> (element=w1238:i32)
                                n544 = flat-sequence {
                                tunnel: w1237 -> [w1244]
                                tunnel: w1238 -> [w1243]
                                tunnel: [w1244] -> w1236
                                tunnel: [w1243] -> w1235
                                tunnel: [w1242] -> w1234
                                tunnel: w1236 -> [w1262]
                                tunnel: w1235 -> [w1259]
                                tunnel: w1234 -> [w1248]
                                frame #0 {
                                n545 = local read "Probe Card Channels"() -> (w1240:i32)
                                n546 = local read "Auto ReCheck"() -> (w1241:bool)
                                n547 = local read "Thresholds:"() -> (w1245:T2)
                                n548 = call "ReCheckStrips.vi"("Probe Card Channels"=w1240, "Auto Re-Check"=w1241, "Thresholds"=w1245, "region in"=w1244, "Number of strips probed"=w1243) -> ("Thresholds copy"=w1242:T17)  [unwired: 6 in]
                                n549 = local write "Thresholds:"(w1242) -> ()
                                }
                                frame #1 {
                                n550 = global read "ProbePlanParams.vi" "ProbePlan Parameters IN"() -> (w1247:T11)
                                n551 = Unbundle By Name(w1247) -> ("Test ProbePoints.Strip length [cm]"=w1246:dbl[])
                                n552 = local read "max scale array"() -> (w1261:i32[])
                                n553 = local read "min scale array"() -> (w1260:i32[])
                                n554 = call "DisplayStriptestData.vi"("Strip Lengths [cm]"=w1246, "min scale array"=w1260, "max scale array"=w1261, "# probed"=w1259, "Display Stats?"=TRUE, "Thresholds:"=w1248, "Region"=w1262) -> ("Defects"=w1254:i32[][], "Resistance [MW]"=w1255:cluster{u32, i32, "Array OUT":dbl[]}, "Capacitance [pF]"=w1257:cluster{u32, i32, "Array OUT":dbl[]}, "Current [nA]"=w1256:cluster{u32, i32, "Array OUT":dbl[]}, "Strip Quality Data"=w1253:T16)
                                n555 = local write "Defects"(w1254) -> ()
                                n556 = local write "Current [nA]"(w1256) -> ()
                                n557 = local write "Capacitance [pF]"(w1257) -> ()
                                n558 = local write "Resistance [MW]"(w1255) -> ()
                                n559 = Unbundle By Name(w1253) -> ("pass Rate in %"=w1252:dbl, "Bad channel list"=w1251:i32[], "No of bad strips"=w1250:i32, "Number of defects per category"=w1249:i32[])
                                n560 = local write "% OK:"(w1252) -> ()
                                n561 = local write "Bad Strip List"(w1251) -> ()
                                n562 = local write "# total defects:"(w1250) -> ()
                                n563 = local write "defect type array"(w1249) -> ()
                                }
                                }
                                }
                              }
                            }
                          }
                          frame #1 {
                            n564 = local write "Auto ReCheck"(FALSE) -> ()
                          }
                        }
                      }
                    }
                  }
                }
                n565 = case shown="True" w1193 {
                  tunnel: w1192 -> [w1264 w1273]
                  tunnel: [w1264 w1273] -> w1190
                  frame False {
                  }
                  frame True {
                    n566 = global read "ProbePlanParams.vi" "ProbePlan Parameters IN"() -> (w1266:T11)
                    n567 = local read "probe points per region"() -> (w1283:i32[])
                    n568 = local read "Region Indices"() -> (w1274:i32[])
                    n569 = Unbundle By Name(w1266) -> ("Test ProbePoints.Strip length [cm]"=w1265:dbl[])
                    n570 = Index Array(array=w1274, index=w1273) -> (element=w1272:i32)
                    n571 = Index Array(array=w1283, index=w1273) -> (element=w1289:i32)
                    n572 = local read "max scale array"() -> (w1284:i32[])
                    n573 = local read "min scale array"() -> (w1285:i32[])
                    n574 = local read "Thresholds:"() -> (w1288:T2)
                    n575 = Index Array(array=w1284, index=w1273) -> (element=w1271:i32)
                    n576 = Index Array(array=w1285, index=w1273) -> (element=w1270:i32)
                    n577 = call "DisplayStriptestData.vi"("Strip Lengths [cm]"=w1265, "min scale array"=w1285, "max scale array"=w1284, "# probed"=w1289, "Display Stats?"=TRUE, "Thresholds:"=w1288, "Region"=w1272) -> ("Defects"=w1286:i32[][], "Resistance [MW]"=w1280:cluster{u32, i32, "Array OUT":dbl[]}, "Capacitance [pF]"=w1281:cluster{u32, i32, "Array OUT":dbl[]}, "Current [nA]"=w1282:cluster{u32, i32, "Array OUT":dbl[]}, "Strip Quality Data"=w1287:T16)
                    n578 = Increment(x=w1271) -> (x+1=w1268:i32)
                    n579 = Increment(x=w1270) -> (x+1=w1269:i32)
                    n580 = local write "Defects"(w1286) -> ()
                    n581 = local write "Current [nA]"(w1282) -> ()
                    n582 = property on="Resistance [MW]" class="WFGraph (strict)"("XScale.Minimum"=w1269) -> ()  [unwired: 2 in, 2 out]
                    n583 = property on="Capacitance [pF]" class="WFGraph (strict)"("XScale.Minimum"=w1269) -> ()  [unwired: 2 in, 2 out]
                    n584 = property on="Defects" class="IntGraph (strict)"("XScale.Minimum"=w1269) -> ()  [unwired: 2 in, 2 out]
                    n585 = property on="Current [nA]" class="WFGraph (strict)"("XScale.Minimum"=w1269) -> ()  [unwired: 2 in, 2 out]
                    n586 = property on="Resistance [MW]" class="WFGraph (strict)"("XScale.Maximum"=w1268) -> ()  [unwired: 2 in, 2 out]
                    n587 = property on="Current [nA]" class="WFGraph (strict)"("XScale.Maximum"=w1268) -> ()  [unwired: 2 in, 2 out]
                    n588 = local write "Capacitance [pF]"(w1281) -> ()
                    n589 = local write "Resistance [MW]"(w1280) -> ()
                    n590 = property on="Capacitance [pF]" class="WFGraph (strict)"("XScale.Maximum"=w1268) -> ()  [unwired: 2 in, 2 out]
                    n591 = Unbundle By Name(w1287) -> ("pass Rate in %"=w1277:dbl, "Bad channel list"=w1275:i32[], "No of bad strips"=w1278:i32, "Number of defects per category"=w1276:i32[])
                    n592 = Increment(x=w1268) -> (x+1=w1267:i32)
                    n593 = local write "% OK:"(w1277) -> ()
                    n594 = local write "Bad Strip List"(w1275) -> ()
                    n595 = local write "# total defects:"(w1278) -> ()
                    n596 = property on="Defects" class="IntGraph (strict)"("XScale.Maximum"=w1267) -> ()  [unwired: 2 in, 2 out]
                    n597 = local write "defect type array"(w1276) -> ()
                  }
                }
                n598 = Or(x="Save Data", y="Quit w/o saving") -> (x .or. y?=w1194:bool)
              }
              n599 = local write "Save Data"("Auto quit &\nswitch off bias") -> ()
            }
            frame #1 {
              n600 = case shown="False" w1290 {
                frame False {
                  # "supply to standby"
                  n601 = global read "QC_MeasurementSetup.vi" "Striptest Measurement Parameters"() -> (w1302:T8)
                  n602 = Unbundle By Name(w1302) -> ("Bias Supply"=w1291:refnum<class "SupplyControl.lvclass">, "Measurement switch"=w1301:refnum<class "Switching.lvclass">)
                  n603 = local read "Current Bias Voltage [V]"() -> (w1295:dbl)
                  n604 = call-dynamic "MatrixSwitch.vi"("Action"=T6."Reset", "Switching in"=w1301) -> ("error out"=w1300:errorcluster)  [unwired: 7 in, 2 out]
                  n605 = call "SupplyRamp.vi"("error in"=w1300, "Requested Voltage"=0.0, "Step Size"=10.0, "Step Delay"=1000, "Supply IN"=w1291, "Starting Voltage"=w1295) -> ("error out"=w1298:errorcluster, "Supply OUT"=w1297:refnum<class "SupplyControl.lvclass">, "Current Voltage"=w1296:dbl)  [unwired: 2 in, 1 out]
                  n606 = call-dynamic "Supply_Stby.vi"("error in (no error)"=w1298, "SupplyControl in"=w1297) -> ()  [unwired: 8 in, 2 out]
                  n607 = local write "Current Bias Voltage [V]"(w1296) -> ()
                }
                frame True {
                }
              }
            }
            frame #2 {
              n608 = case shown="False" w1306 {
                frame False {
                  n609 = global read "QC_MeasurementSetup.vi" "Striptest Measurement Parameters"() -> (w1308:T8)
                  n610 = Unbundle By Name(w1308) -> ("Arduino"=w1313:refnum<class "ArduinoControl.lvclass">)
                  n611 = local read "Temperature Progression"() -> (w1318:T3)
                  n612 = call "ArduinoRead.vi"("Arduino function"=enum16{"T/RH", "Interlock", "Edgesense"}."T/RH", "ArduinoControl in"=w1313) -> ("error out"=w1319:errorcluster, "Temperature [°C]"=w1310:dbl, "ArduinoControl out"=w1320:refnum<class "ArduinoControl.lvclass">)  [unwired: 4 in, 3 out]
                  "Last Temperature [°C]" <- w1310
                  n613 = local read "Run Duration:"() -> (w1315:string)
                  n614 = call "ArduinoClose.vi"("error in (no error)"=w1319, "ArduinoControl in"=w1320) -> ()  [unwired: 8 in, 2 out]
                  n615 = Unbundle(w1318) -> ("Time Array"=w1316:string[], "Temperature Array [°C]"=w1311:dbl[])  [unwired: 1 out]
                  n616 = Build Array (concatenate)(w1316, w1315) -> (w1314:string[])
                  n617 = Build Array (concatenate)(w1311, w1310) -> (w1309:dbl[])
                  n618 = Bundle(cluster=w1318, "Time Array"=w1314, "Temperature Array [°C]"=w1309) -> (w1317:T3)  [unwired: 1 in]
                  n619 = local write "Temperature Progression"(w1317) -> ()
                }
                frame True {
                }
              }
              n620 = local read "# probed"() -> (w1305:i32)
              n621 = Current VI's Path() -> (path=w1303:path)
              n622 = call "SaveJPEG.vi"("Picture No."=w1305, "Test"="Striptest", "File Path Control"=w1303) -> ()  [unwired: 2 out]
              n623 = One Button Dialog(message="Please switch bias off NOW and then open\nprobestation enclosure and raise needle.") -> ()  [unwired: 1 in, 1 out]
            }
            frame #3 {
              n624 = One Button Dialog(message="Please ensure detector bias is OFF!") -> ()  [unwired: 1 in, 1 out]
            }
          }
          n625 = case shown="True" w1177 {
            tunnel: [FALSE w1413] -> w1175
            frame False {
            }
            frame True {
              n626 = Two Button Dialog(message="Are you sure you don't want to save the data?", 1:"Quit" ("F button name (\"Cancel\")"), 2:"Save data" ("T button name (\"OK\")")) -> (T button?=w1413:bool)
            }
          }
          n627 = global read "ProbePlanParams.vi" "ProbePlan Parameters IN"() -> (w1174:T11)
          n628 = Unbundle By Name(w1174) -> ("Test ProbePoints.Regions Enabled"=w1172:bool[], "ProbePlan array"=w1171:T12)
          n629 = Or(x=w1176, y=w1175) -> (x .or. y?=w1165:bool)
          n630 = Array Size(array=w1172) -> (size(s)=w1173:i32)
          n631 = case shown="True" w1165 {
            tunnel: w1173 -> [w1328 w1358]
            tunnel: w1172 -> [w1327 w1357]
            tunnel: w1171 -> [_ w1356]
            tunnel: [w1323 w1354] -> w1168
            tunnel: [w1325 w1352] -> w1167
            tunnel: ["" w1349] -> w1166
            frame False {
              n632 = for {
                N: w1328 -> [_]
                tunnel: w1327 -> [w1332] mode=indexing
                tunnel: [w1331] -> w1326 mode=indexing
                tunnel: [w1330] -> w1324 mode=indexing
                i -> [w1329]
                n633 = case shown="True" w1332 {
                  tunnel: [100.0 w1339] -> w1331
                  tunnel: [TRUE w1338] -> w1330
                  tunnel: w1329 -> [_ w1337]
                  frame False {
                  }
                  frame True {
                    n634 = global read "ProbePlanParams.vi" "ProbePlan Parameters IN"() -> (w1336:T11)
                    n635 = local read "probe points per region"() -> (w1345:i32[])
                    n636 = Unbundle By Name(w1336) -> ("Test ProbePoints.Strip length [cm]"=w1335:dbl[])
                    n637 = Index Array(array=w1345) -> (element=w1341:i32)  [unwired: 1 in]
                    n638 = local read "max scale array"() -> (w1344:i32[])
                    n639 = local read "min scale array"() -> (w1343:i32[])
                    n640 = local read "Thresholds:"() -> (w1347:T2)
                    n641 = call "DisplayStriptestData.vi"("Strip Lengths [cm]"=w1335, "min scale array"=w1343, "max scale array"=w1344, "# probed"=w1341, "Display Stats?"=TRUE, "Thresholds:"=w1347, "Region"=w1337) -> ("Strip Quality Data"=w1342:T16)  [unwired: 4 out]
                    n642 = Unbundle By Name(w1342) -> ("pass Rate in %"=w1339:dbl)
                    n643 = Greater?(x=w1339, y=98.0) -> (0:w1338:bool)
                  }
                }
              }
              n644 = And Array Elements(Boolean array=w1324) -> (logical AND=w1323:bool)
              n645 = Array Max & Min(array=w1326) -> (min value=w1325:dbl)  [unwired: 3 out]
            }
            frame True {
              n646 = for {
                N: w1358 -> [_]
                tunnel: w1357 -> [w1368] mode=indexing
                tunnel: w1356 -> [w1367] mode=indexing
                tunnel: [w1359] -> w1355 mode=indexing
                tunnel: [w1365] -> w1353 mode=indexing
                tunnel: [w1364] -> w1351
                shift-right: [w1363] -> w1348
                shift-left: _ -> [w1360]
                i -> [w1366]
                n647 = case shown="True" w1368 {
                  tunnel: w1366 -> [_ w1381]
                  tunnel: w1367 -> [_ w1380]
                  tunnel: [100.0 w1377] -> w1365
                  tunnel: [w1370 w1376] -> w1364
                  tunnel: [w1370 w1375] -> w1361
                  tunnel: [TRUE w1372] -> w1359
                  frame False {
                    w1370 = ""
                  }
                  frame True {
                    n648 = Unbundle By Name(w1380) -> ("Region"=w1379:string)
                    n649 = flat-sequence {
                      tunnel: w1381 -> [w1383]
                      tunnel: w1379 -> [w1385]
                      tunnel: [w1383] -> w1378
                      tunnel: [w1387] -> w1376
                      tunnel: [w1386] -> w1375
                      tunnel: [w1385] -> w1374
                      tunnel: [w1382] -> w1373
                      tunnel: w1378 -> [w1399]
                      tunnel: [w1404] -> w1377
                      tunnel: w1374 -> [_]
                      tunnel: w1373 -> [w1403]
                      tunnel: [w1398] -> w1372
                      frame #0 {
                        n650 = Concatenate Strings("Saving data for " ("string"), w1385) -> (w1395:string)
                        n651 = local write "Status:"(w1395) -> ()
                        n652 = local read "Temperature Progression"() -> (w1390:T3)
                        n653 = Unbundle By Name(w1390) -> ("Temperature Array [°C]"=w1389:dbl[], "Humidity Array [RH %]"=w1388:dbl[])
                        n654 = call <vilib>:"Std Deviation and Variance.vi"("X"=w1389) -> ("mean"=w1392:dbl)  [unwired: 1 in, 2 out]
                        n655 = call <vilib>:"Std Deviation and Variance.vi"("X"=w1388) -> ("mean"=w1391:dbl)  [unwired: 1 in, 2 out]
                        n656 = call "SaveDataFile.vi"("Temperature"=w1392, "Run uninterrupted?"=FALSE, "Humidity"=w1391, "Sensor Index/\nSegment No."=w1383, "Array Titles"="ProbeplanIndex Current[nA] Capacitance[pF] Resistance[MOhm]", "Strip Segment"=w1385) -> ("Filename OUT"=w1386:string, 6:w1387, "Path + Filename OUT"=w1382:string)  [unwired: 5 in, 2 out]
                      }
                      frame #1 {
                        n657 = global read "ProbePlanParams.vi" "ProbePlan Parameters IN"() -> (w1396:T11)
                        n658 = local read "probe points per region"() -> (w1409:i32[])
                        n659 = Unbundle By Name(w1396) -> ("Test ProbePoints.Strip length [cm]"=w1397:dbl[])
                        n660 = Index Array(array=w1409, index=w1399) -> (element=w1405:i32)
                        n661 = local read "max scale array"() -> (w1408:i32[])
                        n662 = local read "min scale array"() -> (w1407:i32[])
                        n663 = local read "Thresholds:"() -> (w1411:T2)
                        n664 = call "DisplayStriptestData.vi"("Strip Lengths [cm]"=w1397, "min scale array"=w1407, "max scale array"=w1408, "# probed"=w1405, "Display Stats?"=TRUE, "Thresholds:"=w1411, "Region"=w1399) -> ("Strip Quality Data"=w1406:T16)  [unwired: 4 out]
                        n665 = Unbundle By Name(w1406) -> ("pass Rate in %"=w1404:dbl, "No of bad strips"=w1402:i32, "Bad channel list"=w1401:i32[], "Defect description list"=w1400:i32[])
                        n666 = call "CreateDefectFile.vi"("Region"=w1399, "Pass rate"=w1404, "Defect description list"=w1400, "Bad channel array"=w1401, "No of bad strips"=w1402, "Filename IN"=w1403) -> ("passed"=w1398:bool)  [unwired: 4 in, 1 out]
                      }
                    }
                  }
                }
                n667 = call <vilib>:"Space Constant.vi"() -> ("String"=w1362:string)
                n668 = Concatenate Strings(w1360, w1362, w1361) -> (w1363:string)
              }
              n669 = Array Max & Min(array=w1353) -> (min value=w1352:dbl)  [unwired: 3 out]
              n670 = And Array Elements(Boolean array=w1355) -> (logical AND=w1354:bool)
              "Module failed/passed" <- w1354
              n671 = call <vilib>:"Space Constant.vi"() -> ("String"=w1350:string)
              n672 = Concatenate Strings(w1351, w1350, w1348) -> (w1349:string)
            }
          }
          n673 = local read "Temperature Progression"() -> (w1164:T3)
          n674 = Unbundle By Name(w1164) -> ("Temperature Array [°C]"=w1162:dbl[], "Humidity Array [RH %]"=w1163:dbl[])
          n675 = call <vilib>:"Std Deviation and Variance.vi"("X"=w1162) -> ("standard deviation"=w1156:dbl)  [unwired: 1 in, 2 out]
          n676 = call <vilib>:"Std Deviation and Variance.vi"("X"=w1163) -> ("standard deviation"=w1155:dbl)  [unwired: 1 in, 2 out]
          n677 = Greater?(x=w1156, y=5) -> (0:w1153:bool)
          n678 = Greater?(x=w1155, y=10) -> (0:w1154:bool)
          n679 = Select(t="large temperature fluctuations", s=w1153, f=w1159) -> (s? t:f=w1150:string)
          n680 = Select(t="large humidity fluctuations", s=w1154, f=w1159) -> (s? t:f=w1151:string)
          n681 = Concatenate Strings(w1150, "\t", w1151) -> (w1149:string)
          n682 = call "WriteLogFile.vi"("Run uninterrupted?"=FALSE, "Automatic warning"=w1149, "Data File"=w1166, "DUT passed?"=w1168, "Value TechSpec criteria"=w1167, "Files saved?"=w1165) -> ()  [unwired: 5 in, 1 out]
        }
      }
    }
  }
